vi "CRYSet Stimulus Editor Sub Front Panel.vi"(11 "Vi Ref":refnum<vi>) -> ()   [LabVIEW 2013]
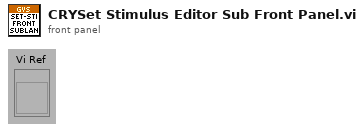
[diagram p1: front panel]
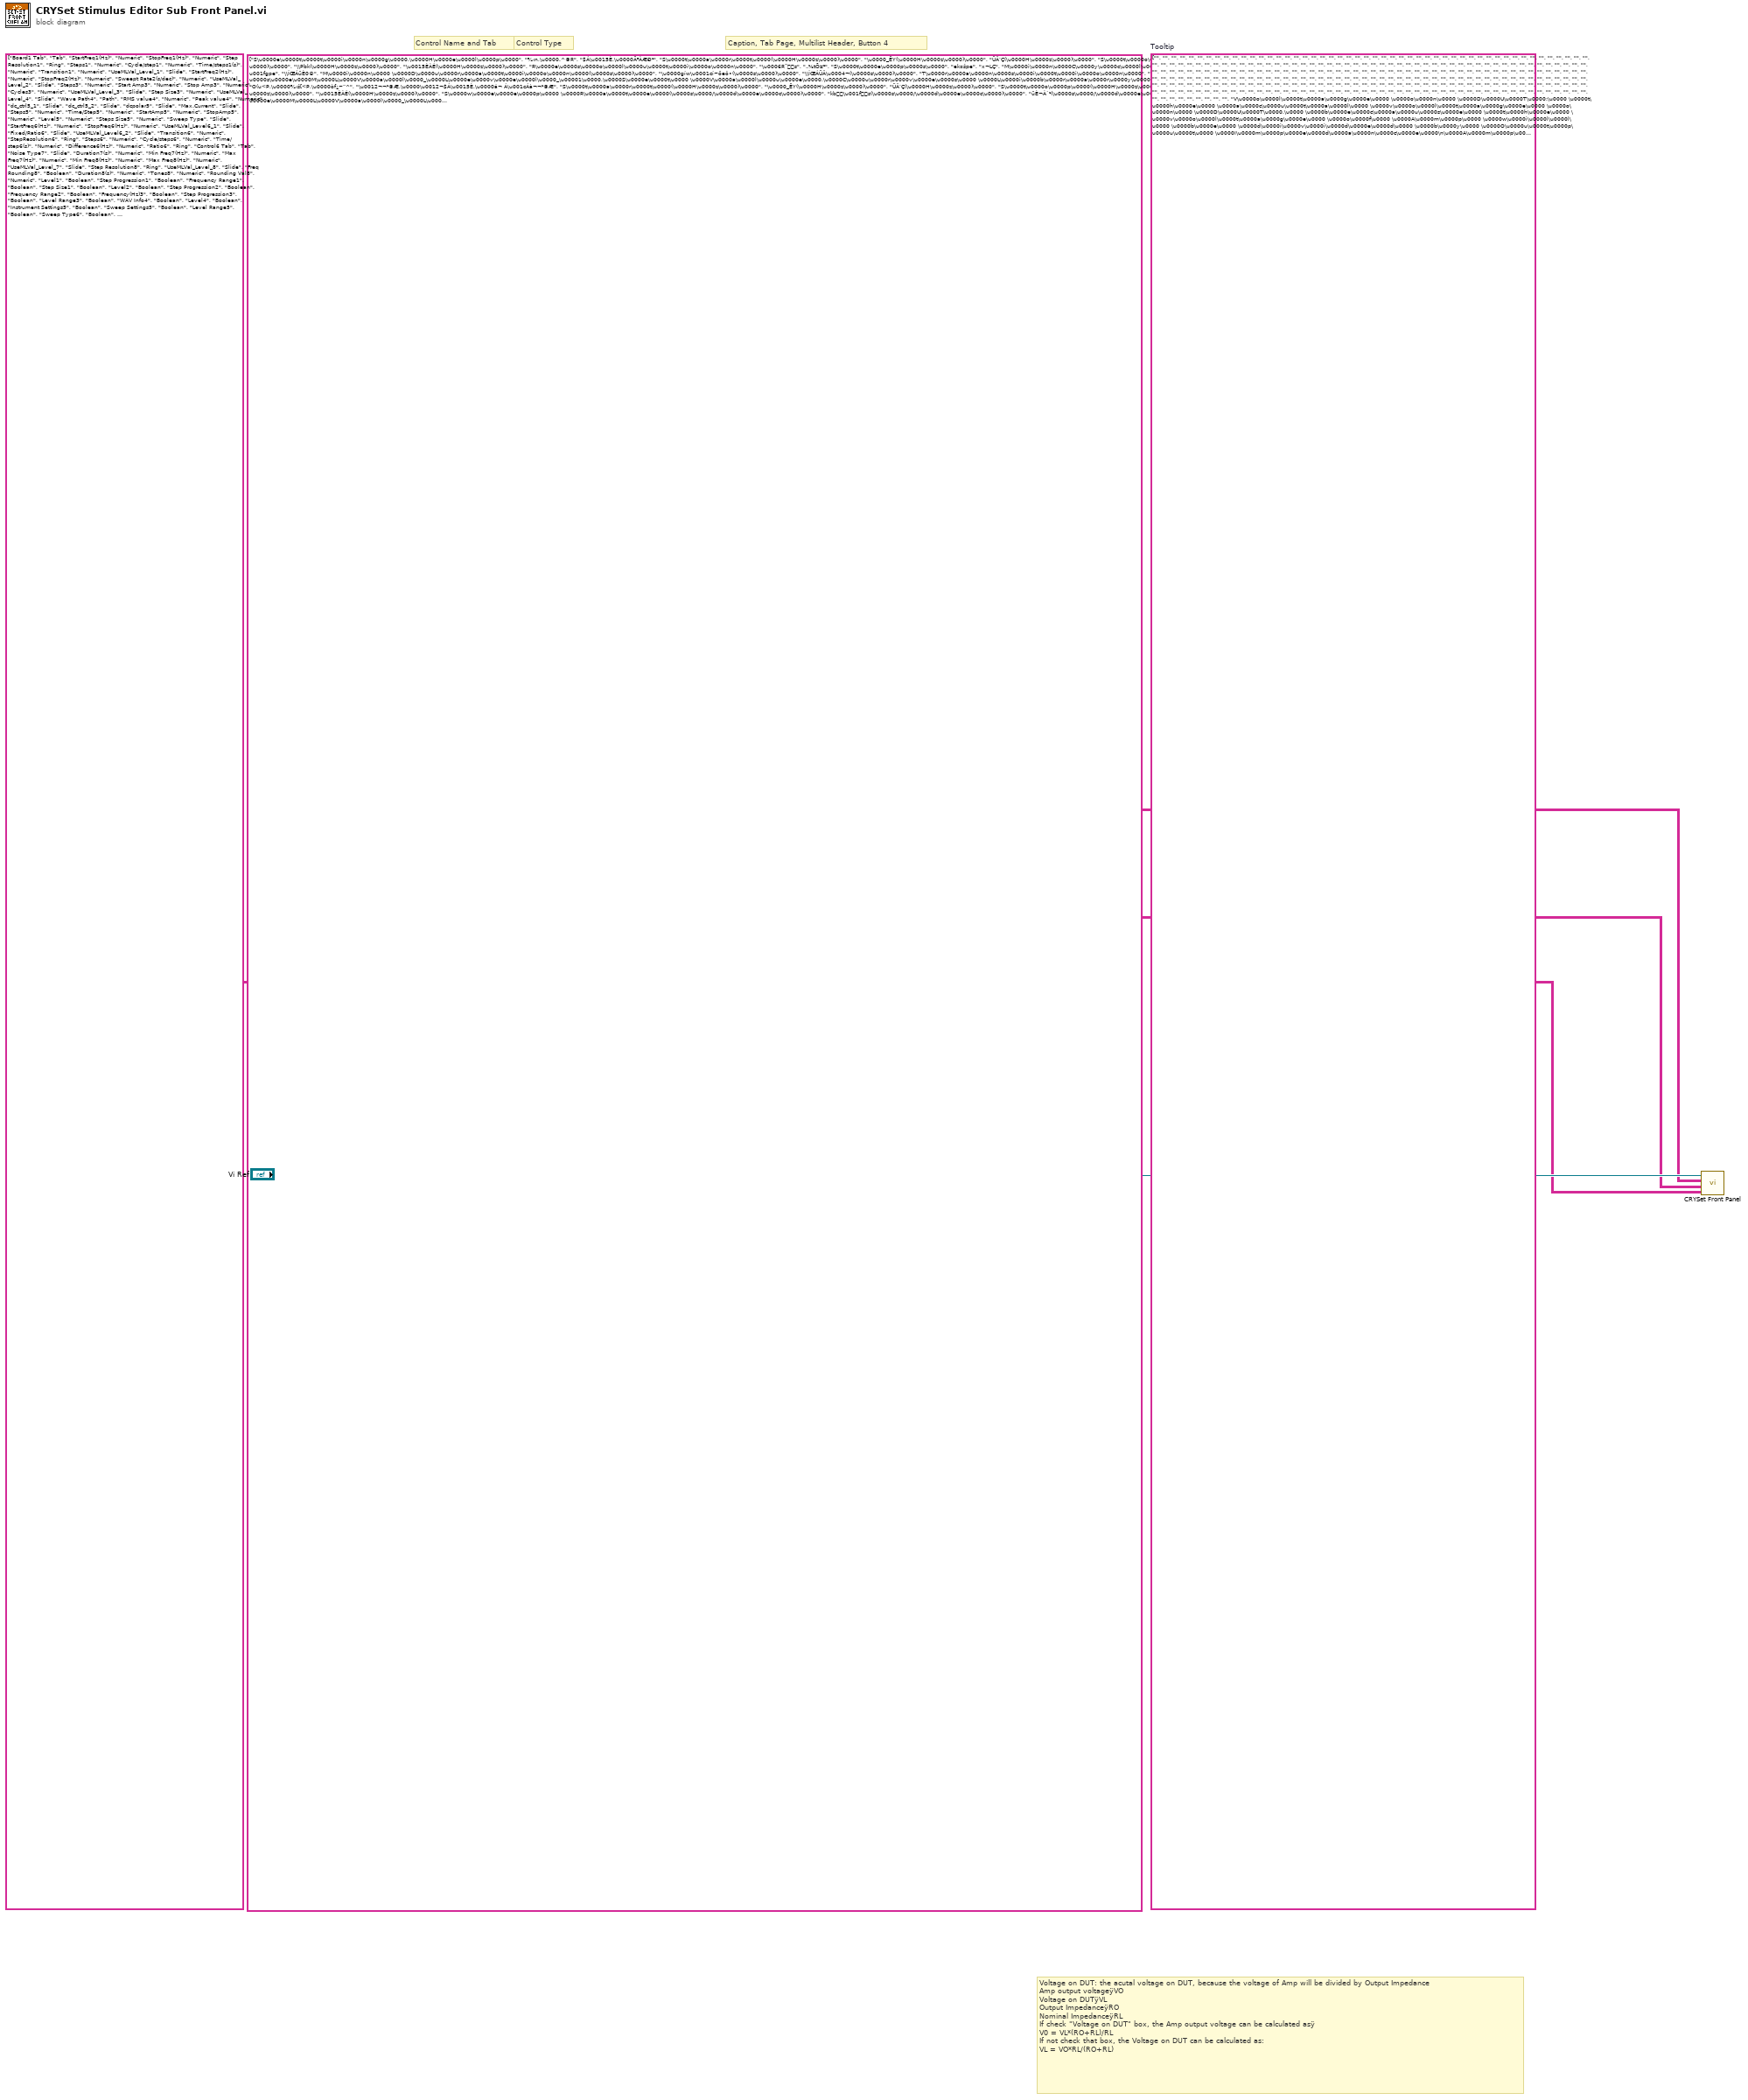
[diagram p0: block diagram]
diagram:
  w1 = string[][] [["", "", ""], ["", "", ""], ["", "", ""], ["", "", ""], ["", "", ""], ["", "", ""], ["", "", ""], ["", "", ""], ["", "", ""], ["", "", ""], ["", "", ""], ["", "", ""], ["", "", ""], ["", "", ""], ["", "", ""], ["", "", ""], ["", "", ""], ["", "", ""], ["", "", ""], ["", "", ""], ["", "", ""], ["", "", ""], ["", "", ""], ["", "", ""], ["", "", ""], ["", "", ""], ["", "", ""], ["", "", ""], ["", "", ""], ["", "", ""], ["", "", ""], ["", "", ""], ["", "", ""], ["", "", ""], ["", "", ""], ["", "", ""], ["", "", ""], ["", "", ""], ["", "", ""], ["", "", ""], ["", "", ""], ["", "", ""], ["", "", ""], ["", "", ""], ["", "", ""], ["", "", ""], ["", "", ""], ["", "", ""], ["", "", ""], ["", "", ""], ["", "", ""], ["", "", ""], ["", "", ""], ["", "", ""], ["", "", ""], ["", "", ""], ["", "", ""], ["", "", ""], ["", "", ""], ["", "", ""], ["", "", ""], ["", "", ""], ["", "", ""], ["", "", ""], ["", "", ""], ["", "", ""], ["", "", ""], ["", "", ""], ["", "", ""], ["", "", ""], ["", "", ""], ["", "", ""], ["", "", ""], ["", "", ""], ["", "", ""], ["", "", ""], ["", "", ""], ["", "", ""], ["", "", ""], ["", "", ""], ["", "", ""], ["", "", ""], ["", "", ""], ["", "", ""], ["", "", ""], ["", "", ""], ["", "", ""], ["", "", ""], ["", "", ""], ["", "", ""], ["", "", ""], ["", "", ""], ["", "", ""], ["", "", ""], ["", "", ""], ["", "", ""], ["", "", ""], ["", "", ""], ["", "", ""], ["", "", ""], ["", "", ""], ["", "", ""], ["", "", ""], ["V\u0000o\u0000l\u0000t\u0000a\u0000g\u0000e\u0000 \u0000o\u0000n\u0000 \u0000D\u0000U\u0000T\u0000:\u0000 \u0000t\u0000h\u0000e\u0000 \u0000a\u0000c\u0000u\u0000t\u0000a\u0000l\u0000 \u0000v\u0000o\u0000l\u0000t\u0000a\u0000g\u0000e\u0000 \u0000o\u0000n\u0000 \u0000D\u0000U\u0000T\u0000,\u0000 \u0000b\u0000e\u0000c\u0000a\u0000u\u0000s\u0000e\u0000 \u0000t\u0000h\u0000e\u0000 \u0000v\u0000o\u0000l\u0000t\u0000a\u0000g\u0000e\u0000 \u0000o\u0000f\u0000 \u0000A\u0000m\u0000p\u0000 \u0000w\u0000i\u0000l\u0000l\u0000 \u0000b\u0000e\u0000 \u0000d\u0000i\u0000v\u0000i\u0000d\u0000e\u0000d\u0000 \u0000b\u0000y\u0000 \u0000O\u0000u\u0000t\u0000p\u0000u\u0000t\u0000 \u0000I\u0000m\u0000p\u0000e\u0000d\u0000a\u0000n\u0000c\u0000e\u0000\n\u0000A\u0000m\u0000p\u0000 \u0000o\u0000u\u0000t\u0000p\u0000u\u0000t\u0000 \u0000v\u0000o\u0000l\u0000t\u0000a\u0000g\u0000e\u0000\u001aÿV\u0000O\u0000\n\u0000V\u0000o\u0000l\u0000t\u0000a\u0000g\u0000e\u0000 \u0000o\u0000n\u0000 \u0000D\u0000U\u0000T\u0000\u001aÿV\u0000L\u0000\n\u0000O\u0000u\u0000t\u0000p\u0000u\u0000t\u0000 \u0000I\u0000m\u0000p\u0000e\u0000d\u0000a\u0000n\u0000c\u0000e\u0000\u001aÿR\u0000O\u0000\n\u0000N\u0000o\u0000m\u0000i\u0000n\u0000a\u0000l\u0000 \u0000I\u0000m\u0000p\u0000e\u0000d\u0000a\u0000n\u0000c\u0000e\u0000\u001aÿR\u0000L\u0000\n\u0000I\u0000f\u0000 \u0000c\u0000h\u0000e\u0000c\u0000k\u0000 \u0000\"\u0000V\u0000o\u0000l\u0000t\u0000a\u0000g\u0000e\u0000 \u0000o\u0000n\u0000 \u0000D\u0000U\u0000T\u0000\"\u0000 \u0000b\u0000o\u0000x\u0000,\u0000 \u0000t\u0000h\u0000e\u0000 \u0000A\u0000m\u0000p\u0000 \u0000o\u0000u\u0000t\u0000p\u0000u\u0000t\u0000 \u0000v\u0000o\u0000l\u0000t\u0000a\u0000g\u0000e\u0000 \u0000c\u0000a\u0000n\u0000 \u0000b\u0000e\u0000 \u0000c\u0000a\u0000l\u0000c\u0000u\u0000l\u0000a\u0000t\u0000e\u0000d\u0000 \u0000a\u0000s\u0000\u001aÿ\n\u0000V\u00000\u0000 \u0000=\u0000 \u0000V\u0000L\u0000*\u0000(\u0000R\u0000O\u0000+\u0000R\u0000L\u0000)\u0000/\u0000R\u0000L\u0000\n\u0000I\u0000f\u0000 \u0000n\u0000o\u0000t\u0000 \u0000c\u0000h\u0000e\u0000c\u0000k\u0000 \u0000t\u0000h\u0000a\u0000t\u0000 \u0000...", "hVöN$Nïz5uS\u001aÿR>eúQv5uS\fÿÏ~ÇúQ;b\u0006RS\u000eT\fÿ(W«KmhVöN$Nïzv[E5uS\u00020\n\u0000\n\u0000R>eúQ5uS\u001aÿV\u0000O\u0000\n\u0000hVöN$Nïz5uS\u001aÿV\u0000L\u0000\n\u0000úQ;b\u001aÿR\u0000O\u0000\n\u0000\u0007hðy;b\u001aÿR\u0000L\u0000\n\u0000\n\u0000å\t-NhVöN$Nïz5uS\fÿ\u0019RR>eúQ5uS:N\u001aÿ\n\u0000V\u00000\u0000 \u0000=\u0000 \u0000V\u0000L\u0000*\u0000(\u0000R\u0000O\u0000+\u0000R\u0000L\u0000)\u0000/\u0000R\u0000L\u0000\n\u0000\n\u0000å\rN\t-N\fÿ\u0019RhVöN$Nïz5uS:N\u001aÿ\n\u0000V\u0000L\u0000 \u0000=\u0000 \u0000V\u0000O\u0000*\u0000R\u0000L\u0000/\u0000(\u0000R\u0000O\u0000+\u0000R\u0000L\u0000)\u0000", "V\u0000o\u0000l\u0000t\u0000a\u0000g\u0000e\u0000 \u0000o\u0000n\u0000 \u0000D\u0000U\u0000T\u0000:\u0000 \u0000t\u0000h\u0000e\u0000 \u0000a\u0000c\u0000u\u0000t\u0000a\u0000l\u0000 \u0000v\u0000o\u0000l\u0000t\u0000a\u0000g\u0000e\u0000 \u0000o\u0000n\u0000 \u0000D\u0000U\u0000T\u0000,\u0000 \u0000b\u0000e\u0000c\u0000a\u0000u\u0000s\u0000e\u0000 \u0000t\u0000h\u0000e\u0000 \u0000v\u0000o\u0000l\u0000t\u0000a\u0000g\u0000e\u0000 \u0000o\u0000f\u0000 \u0000A\u0000m\u0000p\u0000 \u0000w\u0000i\u0000l\u0000l\u0000 \u0000b\u0000e\u0000 \u0000d\u0000i\u0000v\u0000i\u0000d\u0000e\u0000d\u0000 \u0000b\u0000y\u0000 \u0000O\u0000u\u0000t\u0000p\u0000u\u0000t\u0000 \u0000I\u0000m\u0000p\u0000e\u0000d\u0000a\u0000n\u0000c\u0000e\u0000\n\u0000A\u0000m\u0000p\u0000 \u0000o\u0000u\u0000t\u0000p\u0000u\u0000t\u0000 \u0000v\u0000o\u0000l\u0000t\u0000a\u0000g\u0000e\u0000\u001aÿV\u0000O\u0000\n\u0000V\u0000o\u0000l\u0000t\u0000a\u0000g\u0000e\u0000 \u0000o\u0000n\u0000 \u0000D\u0000U\u0000T\u0000\u001aÿV\u0000L\u0000\n\u0000O\u0000u\u0000t\u0000p\u0000u\u0000t\u0000 \u0000I\u0000m\u0000p\u0000e\u0000d\u0000a\u0000n\u0000c\u0000e\u0000\u001aÿR\u0000O\u0000\n\u0000N\u0000o\u0000m\u0000i\u0000n\u0000a\u0000l\u0000 \u0000I\u0000m\u0000p\u0000e\u0000d\u0000a\u0000n\u0000c\u0000e\u0000\u001aÿR\u0000L\u0000\n\u0000I\u0000f\u0000 \u0000c\u0000h\u0000e\u0000c\u0000k\u0000 \u0000\"\u0000V\u0000o\u0000l\u0000t\u0000a\u0000g\u0000e\u0000 \u0000o\u0000n\u0000 \u0000D\u0000U\u0000T\u0000\"\u0000 \u0000b\u0000o\u0000x\u0000,\u0000 \u0000t\u0000h\u0000e\u0000 \u0000A\u0000m\u0000p\u0000 \u0000o\u0000u\u0000t\u0000p\u0000u\u0000t\u0000 \u0000v\u0000o\u0000l\u0000t\u0000a\u0000g\u0000e\u0000 \u0000c\u0000a\u0000n\u0000 \u0000b\u0000e\u0000 \u0000c\u0000a\u0000l\u0000c\u0000u\u0000l\u0000a\u0000t\u0000e\u0000d\u0000 \u0000a\u0000s\u0000\u001aÿ\n\u0000V\u00000\u0000 \u0000=\u0000 \u0000V\u0000L\u0000*\u0000(\u0000R\u0000O\u0000+\u0000R\u0000L\u0000)\u0000/\u0000R\u0000L\u0000\n\u0000I\u0000f\u0000 \u0000n\u0000o\u0000t\u0000 \u0000c\u0000h\u0000e\u0000c\u0000k\u0000 \u0000t\u0000h\u0000a\u0000t\u0000 \u0000..."], ["", "", ""], ["", "", ""], ["V\u0000o\u0000l\u0000t\u0000a\u0000g\u0000e\u0000 \u0000o\u0000n\u0000 \u0000D\u0000U\u0000T\u0000:\u0000 \u0000t\u0000h\u0000e\u0000 \u0000a\u0000c\u0000u\u0000t\u0000a\u0000l\u0000 \u0000v\u0000o\u0000l\u0000t\u0000a\u0000g\u0000e\u0000 \u0000o\u0000n\u0000 \u0000D\u0000U\u0000T\u0000,\u0000 \u0000b\u0000e\u0000c\u0000a\u0000u\u0000s\u0000e\u0000 \u0000t\u0000h\u0000e\u0000 \u0000v\u0000o\u0000l\u0000t\u0000a\u0000g\u0000e\u0000 \u0000o\u0000f\u0000 \u0000A\u0000m\u0000p\u0000 \u0000w\u0000i\u0000l\u0000l\u0000 \u0000b\u0000e\u0000 \u0000d\u0000i\u0000v\u0000i\u0000d\u0000e\u0000d\u0000 \u0000b\u0000y\u0000 \u0000O\u0000u\u0000t\u0000p\u0000u\u0000t\u0000 \u0000I\u0000m\u0000p\u0000e\u0000d\u0000a\u0000n\u0000c\u0000e\u0000\n\u0000A\u0000m\u0000p\u0000 \u0000o\u0000u\u0000t\u0000p\u0000u\u0000t\u0000 \u0000v\u0000o\u0000l\u0000t\u0000a\u0000g\u0000e\u0000\u001aÿV\u0000O\u0000\n\u0000V\u0000o\u0000l\u0000t\u0000a\u0000g\u0000e\u0000 \u0000o\u0000n\u0000 \u0000D\u0000U\u0000T\u0000\u001aÿV\u0000L\u0000\n\u0000O\u0000u\u0000t\u0000p\u0000u\u0000t\u0000 \u0000I\u0000m\u0000p\u0000e\u0000d\u0000a\u0000n\u0000c\u0000e\u0000\u001aÿR\u0000O\u0000\n\u0000N\u0000o\u0000m\u0000i\u0000n\u0000a\u0000l\u0000 \u0000I\u0000m\u0000p\u0000e\u0000d\u0000a\u0000n\u0000c\u0000e\u0000\u001aÿR\u0000L\u0000\n\u0000I\u0000f\u0000 \u0000c\u0000h\u0000e\u0000c\u0000k\u0000 \u0000\"\u0000V\u0000o\u0000l\u0000t\u0000a\u0000g\u0000e\u0000 \u0000o\u0000n\u0000 \u0000D\u0000U\u0000T\u0000\"\u0000 \u0000b\u0000o\u0000x\u0000,\u0000 \u0000t\u0000h\u0000e\u0000 \u0000A\u0000m\u0000p\u0000 \u0000o\u0000u\u0000t\u0000p\u0000u\u0000t\u0000 \u0000v\u0000o\u0000l\u0000t\u0000a\u0000g\u0000e\u0000 \u0000c\u0000a\u0000n\u0000 \u0000b\u0000e\u0000 \u0000c\u0000a\u0000l\u0000c\u0000u\u0000l\u0000a\u0000t\u0000e\u0000d\u0000 \u0000a\u0000s\u0000\u001aÿ\n\u0000V\u00000\u0000 \u0000=\u0000 \u0000V\u0000L\u0000*\u0000(\u0000R\u0000O\u0000+\u0000R\u0000L\u0000)\u0000/\u0000R\u0000L\u0000\n\u0000I\u0000f\u0000 \u0000n\u0000o\u0000t\u0000 \u0000c\u0000h\u0000e\u0000c\u0000k\u0000 \u0000t\u0000h\u0000a\u0000t\u0000 \u0000...", "hVöN$Nïz5uS\u001aÿR>eúQv5uS\fÿÏ~ÇúQ;b\u0006RS\u000eT\fÿ(W«KmhVöN$Nïzv[E5uS\u00020\n\u0000\n\u0000R>eúQ5uS\u001aÿV\u0000O\u0000\n\u0000hVöN$Nïz5uS\u001aÿV\u0000L\u0000\n\u0000úQ;b\u001aÿR\u0000O\u0000\n\u0000\u0007hðy;b\u001aÿR\u0000L\u0000\n\u0000\n\u0000å\t-NhVöN$Nïz5uS\fÿ\u0019RR>eúQ5uS:N\u001aÿ\n\u0000V\u00000\u0000 \u0000=\u0000 \u0000V\u0000L\u0000*\u0000(\u0000R\u0000O\u0000+\u0000R\u0000L\u0000)\u0000/\u0000R\u0000L\u0000\n\u0000\n\u0000å\rN\t-N\fÿ\u0019RhVöN$Nïz5uS:N\u001aÿ\n\u0000V\u0000L\u0000 \u0000=\u0000 \u0000V\u0000O\u0000*\u0000R\u0000L\u0000/\u0000(\u0000R\u0000O\u0000+\u0000R\u0000L\u0000)\u0000", "V\u0000o\u0000l\u0000t\u0000a\u0000g\u0000e\u0000 \u0000o\u0000n\u0000 \u0000D\u0000U\u0000T\u0000:\u0000 \u0000t\u0000h\u0000e\u0000 \u0000a\u0000c\u0000u\u0000t\u0000a\u0000l\u0000 \u0000v\u0000o\u0000l\u0000t\u0000a\u0000g\u0000e\u0000 \u0000o\u0000n\u0000 \u0000D\u0000U\u0000T\u0000,\u0000 \u0000b\u0000e\u0000c\u0000a\u0000u\u0000s\u0000e\u0000 \u0000t\u0000h\u0000e\u0000 \u0000v\u0000o\u0000l\u0000t\u0000a\u0000g\u0000e\u0000 \u0000o\u0000f\u0000 \u0000A\u0000m\u0000p\u0000 \u0000w\u0000i\u0000l\u0000l\u0000 \u0000b\u0000e\u0000 \u0000d\u0000i\u0000v\u0000i\u0000d\u0000e\u0000d\u0000 \u0000b\u0000y\u0000 \u0000O\u0000u\u0000t\u0000p\u0000u\u0000t\u0000 \u0000I\u0000m\u0000p\u0000e\u0000d\u0000a\u0000n\u0000c\u0000e\u0000\n\u0000A\u0000m\u0000p\u0000 \u0000o\u0000u\u0000t\u0000p\u0000u\u0000t\u0000 \u0000v\u0000o\u0000l\u0000t\u0000a\u0000g\u0000e\u0000\u001aÿV\u0000O\u0000\n\u0000V\u0000o\u0000l\u0000t\u0000a\u0000g\u0000e\u0000 \u0000o\u0000n\u0000 \u0000D\u0000U\u0000T\u0000\u001aÿV\u0000L\u0000\n\u0000O\u0000u\u0000t\u0000p\u0000u\u0000t\u0000 \u0000I\u0000m\u0000p\u0000e\u0000d\u0000a\u0000n\u0000c\u0000e\u0000\u001aÿR\u0000O\u0000\n\u0000N\u0000o\u0000m\u0000i\u0000n\u0000a\u0000l\u0000 \u0000I\u0000m\u0000p\u0000e\u0000d\u0000a\u0000n\u0000c\u0000e\u0000\u001aÿR\u0000L\u0000\n\u0000I\u0000f\u0000 \u0000c\u0000h\u0000e\u0000c\u0000k\u0000 \u0000\"\u0000V\u0000o\u0000l\u0000t\u0000a\u0000g\u0000e\u0000 \u0000o\u0000n\u0000 \u0000D\u0000U\u0000T\u0000\"\u0000 \u0000b\u0000o\u0000x\u0000,\u0000 \u0000t\u0000h\u0000e\u0000 \u0000A\u0000m\u0000p\u0000 \u0000o\u0000u\u0000t\u0000p\u0000u\u0000t\u0000 \u0000v\u0000o\u0000l\u0000t\u0000a\u0000g\u0000e\u0000 \u0000c\u0000a\u0000n\u0000 \u0000b\u0000e\u0000 \u0000c\u0000a\u0000l\u0000c\u0000u\u0000l\u0000a\u0000t\u0000e\u0000d\u0000 \u0000a\u0000s\u0000\u001aÿ\n\u0000V\u00000\u0000 \u0000=\u0000 \u0000V\u0000L\u0000*\u0000(\u0000R\u0000O\u0000+\u0000R\u0000L\u0000)\u0000/\u0000R\u0000L\u0000\n\u0000I\u0000f\u0000 \u0000n\u0000o\u0000t\u0000 \u0000c\u0000h\u0000e\u0000c\u0000k\u0000 \u0000t\u0000h\u0000a\u0000t\u0000 \u0000..."], ["", "", ""], ["", "", ""], ["V\u0000o\u0000l\u0000t\u0000a\u0000g\u0000e\u0000 \u0000o\u0000n\u0000 \u0000D\u0000U\u0000T\u0000:\u0000 \u0000t\u0000h\u0000e\u0000 \u0000a\u0000c\u0000u\u0000t\u0000a\u0000l\u0000 \u0000v\u0000o\u0000l\u0000t\u0000a\u0000g\u0000e\u0000 \u0000o\u0000n\u0000 \u0000D\u0000U\u0000T\u0000,\u0000 \u0000b\u0000e\u0000c\u0000a\u0000u\u0000s\u0000e\u0000 \u0000t\u0000h\u0000e\u0000 \u0000v\u0000o\u0000l\u0000t\u0000a\u0000g\u0000e\u0000 \u0000o\u0000f\u0000 \u0000A\u0000m\u0000p\u0000 \u0000w\u0000i\u0000l\u0000l\u0000 \u0000b\u0000e\u0000 \u0000d\u0000i\u0000v\u0000i\u0000d\u0000e\u0000d\u0000 \u0000b\u0000y\u0000 \u0000O\u0000u\u0000t\u0000p\u0000u\u0000t\u0000 \u0000I\u0000m\u0000p\u0000e\u0000d\u0000a\u0000n\u0000c\u0000e\u0000\n\u0000A\u0000m\u0000p\u0000 \u0000o\u0000u\u0000t\u0000p\u0000u\u0000t\u0000 \u0000v\u0000o\u0000l\u0000t\u0000a\u0000g\u0000e\u0000\u001aÿV\u0000O\u0000\n\u0000V\u0000o\u0000l\u0000t\u0000a\u0000g\u0000e\u0000 \u0000o\u0000n\u0000 \u0000D\u0000U\u0000T\u0000\u001aÿV\u0000L\u0000\n\u0000O\u0000u\u0000t\u0000p\u0000u\u0000t\u0000 \u0000I\u0000m\u0000p\u0000e\u0000d\u0000a\u0000n\u0000c\u0000e\u0000\u001aÿR\u0000O\u0000\n\u0000N\u0000o\u0000m\u0000i\u0000n\u0000a\u0000l\u0000 \u0000I\u0000m\u0000p\u0000e\u0000d\u0000a\u0000n\u0000c\u0000e\u0000\u001aÿR\u0000L\u0000\n\u0000I\u0000f\u0000 \u0000c\u0000h\u0000e\u0000c\u0000k\u0000 \u0000\"\u0000V\u0000o\u0000l\u0000t\u0000a\u0000g\u0000e\u0000 \u0000o\u0000n\u0000 \u0000D\u0000U\u0000T\u0000\"\u0000 \u0000b\u0000o\u0000x\u0000,\u0000 \u0000t\u0000h\u0000e\u0000 \u0000A\u0000m\u0000p\u0000 \u0000o\u0000u\u0000t\u0000p\u0000u\u0000t\u0000 \u0000v\u0000o\u0000l\u0000t\u0000a\u0000g\u0000e\u0000 \u0000c\u0000a\u0000n\u0000 \u0000b\u0000e\u0000 \u0000c\u0000a\u0000l\u0000c\u0000u\u0000l\u0000a\u0000t\u0000e\u0000d\u0000 \u0000a\u0000s\u0000\u001aÿ\n\u0000V\u00000\u0000 \u0000=\u0000 \u0000V\u0000L\u0000*\u0000(\u0000R\u0000O\u0000+\u0000R\u0000L\u0000)\u0000/\u0000R\u0000L\u0000\n\u0000I\u0000f\u0000 \u0000n\u0000o\u0000t\u0000 \u0000c\u0000h\u0000e\u0000c\u0000k\u0000 \u0000t\u0000h\u0000a\u0000t\u0000 \u0000...", "hVöN$Nïz5uS\u001aÿR>eúQv5uS\fÿÏ~ÇúQ;b\u0006RS\u000eT\fÿ(W«KmhVöN$Nïzv[E5uS\u00020\n\u0000\n\u0000R>eúQ5uS\u001aÿV\u0000O\u0000\n\u0000hVöN$Nïz5uS\u001aÿV\u0000L\u0000\n\u0000úQ;b\u001aÿR\u0000O\u0000\n\u0000\u0007hðy;b\u001aÿR\u0000L\u0000\n\u0000\n\u0000å\t-NhVöN$Nïz5uS\fÿ\u0019RR>eúQ5uS:N\u001aÿ\n\u0000V\u00000\u0000 \u0000=\u0000 \u0000V\u0000L\u0000*\u0000(\u0000R\u0000O\u0000+\u0000R\u0000L\u0000)\u0000/\u0000R\u0000L\u0000\n\u0000\n\u0000å\rN\t-N\fÿ\u0019RhVöN$Nïz5uS:N\u001aÿ\n\u0000V\u0000L\u0000 \u0000=\u0000 \u0000V\u0000O\u0000*\u0000R\u0000L\u0000/\u0000(\u0000R\u0000O\u0000+\u0000R\u0000L\u0000)\u0000", "V\u0000o\u0000l\u0000t\u0000a\u0000g\u0000e\u0000 \u0000o\u0000n\u0000 \u0000D\u0000U\u0000T\u0000:\u0000 \u0000t\u0000h\u0000e\u0000 \u0000a\u0000c\u0000u\u0000t\u0000a\u0000l\u0000 \u0000v\u0000o\u0000l\u0000t\u0000a\u0000g\u0000e\u0000 \u0000o\u0000n\u0000 \u0000D\u0000U\u0000T\u0000,\u0000 \u0000b\u0000e\u0000c\u0000a\u0000u\u0000s\u0000e\u0000 \u0000t\u0000h\u0000e\u0000 \u0000v\u0000o\u0000l\u0000t\u0000a\u0000g\u0000e\u0000 \u0000o\u0000f\u0000 \u0000A\u0000m\u0000p\u0000 \u0000w\u0000i\u0000l\u0000l\u0000 \u0000b\u0000e\u0000 \u0000d\u0000i\u0000v\u0000i\u0000d\u0000e\u0000d\u0000 \u0000b\u0000y\u0000 \u0000O\u0000u\u0000t\u0000p\u0000u\u0000t\u0000 \u0000I\u0000m\u0000p\u0000e\u0000d\u0000a\u0000n\u0000c\u0000e\u0000\n\u0000A\u0000m\u0000p\u0000 \u0000o\u0000u\u0000t\u0000p\u0000u\u0000t\u0000 \u0000v\u0000o\u0000l\u0000t\u0000a\u0000g\u0000e\u0000\u001aÿV\u0000O\u0000\n\u0000V\u0000o\u0000l\u0000t\u0000a\u0000g\u0000e\u0000 \u0000o\u0000n\u0000 \u0000D\u0000U\u0000T\u0000\u001aÿV\u0000L\u0000\n\u0000O\u0000u\u0000t\u0000p\u0000u\u0000t\u0000 \u0000I\u0000m\u0000p\u0000e\u0000d\u0000a\u0000n\u0000c\u0000e\u0000\u001aÿR\u0000O\u0000\n\u0000N\u0000o\u0000m\u0000i\u0000n\u0000a\u0000l\u0000 \u0000I\u0000m\u0000p\u0000e\u0000d\u0000a\u0000n\u0000c\u0000e\u0000\u001aÿR\u0000L\u0000\n\u0000I\u0000f\u0000 \u0000c\u0000h\u0000e\u0000c\u0000k\u0000 \u0000\"\u0000V\u0000o\u0000l\u0000t\u0000a\u0000g\u0000e\u0000 \u0000o\u0000n\u0000 \u0000D\u0000U\u0000T\u0000\"\u0000 \u0000b\u0000o\u0000x\u0000,\u0000 \u0000t\u0000h\u0000e\u0000 \u0000A\u0000m\u0000p\u0000 \u0000o\u0000u\u0000t\u0000p\u0000u\u0000t\u0000 \u0000v\u0000o\u0000l\u0000t\u0000a\u0000g\u0000e\u0000 \u0000c\u0000a\u0000n\u0000 \u0000b\u0000e\u0000 \u0000c\u0000a\u0000l\u0000c\u0000u\u0000l\u0000a\u0000t\u0000e\u0000d\u0000 \u0000a\u0000s\u0000\u001aÿ\n\u0000V\u00000\u0000 \u0000=\u0000 \u0000V\u0000L\u0000*\u0000(\u0000R\u0000O\u0000+\u0000R\u0000L\u0000)\u0000/\u0000R\u0000L\u0000\n\u0000I\u0000f\u0000 \u0000n\u0000o\u0000t\u0000 \u0000c\u0000h\u0000e\u0000c\u0000k\u0000 \u0000t\u0000h\u0000a\u0000t\u0000 \u0000..."], ["", "", ""], ["", "", ""], ["V\u0000o\u0000l\u0000t\u0000a\u0000g\u0000e\u0000 \u0000o\u0000n\u0000 \u0000D\u0000U\u0000T\u0000:\u0000 \u0000t\u0000h\u0000e\u0000 \u0000a\u0000c\u0000u\u0000t\u0000a\u0000l\u0000 \u0000v\u0000o\u0000l\u0000t\u0000a\u0000g\u0000e\u0000 \u0000o\u0000n\u0000 \u0000D\u0000U\u0000T\u0000,\u0000 \u0000b\u0000e\u0000c\u0000a\u0000u\u0000s\u0000e\u0000 \u0000t\u0000h\u0000e\u0000 \u0000v\u0000o\u0000l\u0000t\u0000a\u0000g\u0000e\u0000 \u0000o\u0000f\u0000 \u0000A\u0000m\u0000p\u0000 \u0000w\u0000i\u0000l\u0000l\u0000 \u0000b\u0000e\u0000 \u0000d\u0000i\u0000v\u0000i\u0000d\u0000e\u0000d\u0000 \u0000b\u0000y\u0000 \u0000O\u0000u\u0000t\u0000p\u0000u\u0000t\u0000 \u0000I\u0000m\u0000p\u0000e\u0000d\u0000a\u0000n\u0000c\u0000e\u0000\n\u0000A\u0000m\u0000p\u0000 \u0000o\u0000u\u0000t\u0000p\u0000u\u0000t\u0000 \u0000v\u0000o\u0000l\u0000t\u0000a\u0000g\u0000e\u0000\u001aÿV\u0000O\u0000\n\u0000V\u0000o\u0000l\u0000t\u0000a\u0000g\u0000e\u0000 \u0000o\u0000n\u0000 \u0000D\u0000U\u0000T\u0000\u001aÿV\u0000L\u0000\n\u0000O\u0000u\u0000t\u0000p\u0000u\u0000t\u0000 \u0000I\u0000m\u0000p\u0000e\u0000d\u0000a\u0000n\u0000c\u0000e\u0000\u001aÿR\u0000O\u0000\n\u0000N\u0000o\u0000m\u0000i\u0000n\u0000a\u0000l\u0000 \u0000I\u0000m\u0000p\u0000e\u0000d\u0000a\u0000n\u0000c\u0000e\u0000\u001aÿR\u0000L\u0000\n\u0000I\u0000f\u0000 \u0000c\u0000h\u0000e\u0000c\u0000k\u0000 \u0000\"\u0000V\u0000o\u0000l\u0000t\u0000a\u0000g\u0000e\u0000 \u0000o\u0000n\u0000 \u0000D\u0000U\u0000T\u0000\"\u0000 \u0000b\u0000o\u0000x\u0000,\u0000 \u0000t\u0000h\u0000e\u0000 \u0000A\u0000m\u0000p\u0000 \u0000o\u0000u\u0000t\u0000p\u0000u\u0000t\u0000 \u0000v\u0000o\u0000l\u0000t\u0000a\u0000g\u0000e\u0000 \u0000c\u0000a\u0000n\u0000 \u0000b\u0000e\u0000 \u0000c\u0000a\u0000l\u0000c\u0000u\u0000l\u0000a\u0000t\u0000e\u0000d\u0000 \u0000a\u0000s\u0000\u001aÿ\n\u0000V\u00000\u0000 \u0000=\u0000 \u0000V\u0000L\u0000*\u0000(\u0000R\u0000O\u0000+\u0000R\u0000L\u0000)\u0000/\u0000R\u0000L\u0000\n\u0000I\u0000f\u0000 \u0000n\u0000o\u0000t\u0000 \u0000c\u0000h\u0000e\u0000c\u0000k\u0000 \u0000t\u0000h\u0000a\u0000t\u0000 \u0000...", "hVöN$Nïz5uS\u001aÿR>eúQv5uS\fÿÏ~ÇúQ;b\u0006RS\u000eT\fÿ(W«KmhVöN$Nïzv[E5uS\u00020\n\u0000\n\u0000R>eúQ5uS\u001aÿV\u0000O\u0000\n\u0000hVöN$Nïz5uS\u001aÿV\u0000L\u0000\n\u0000úQ;b\u001aÿR\u0000O\u0000\n\u0000\u0007hðy;b\u001aÿR\u0000L\u0000\n\u0000\n\u0000å\t-NhVöN$Nïz5uS\fÿ\u0019RR>eúQ5uS:N\u001aÿ\n\u0000V\u00000\u0000 \u0000=\u0000 \u0000V\u0000L\u0000*\u0000(\u0000R\u0000O\u0000+\u0000R\u0000L\u0000)\u0000/\u0000R\u0000L\u0000\n\u0000\n\u0000å\rN\t-N\fÿ\u0019RhVöN$Nïz5uS:N\u001aÿ\n\u0000V\u0000L\u0000 \u0000=\u0000 \u0000V\u0000O\u0000*\u0000R\u0000L\u0000/\u0000(\u0000R\u0000O\u0000+\u0000R\u0000L\u0000)\u0000", "V\u0000o\u0000l\u0000t\u0000a\u0000g\u0000e\u0000 \u0000o\u0000n\u0000 \u0000D\u0000U\u0000T\u0000:\u0000 \u0000t\u0000h\u0000e\u0000 \u0000a\u0000c\u0000u\u0000t\u0000a\u0000l\u0000 \u0000v\u0000o\u0000l\u0000t\u0000a\u0000g\u0000e\u0000 \u0000o\u0000n\u0000 \u0000D\u0000U\u0000T\u0000,\u0000 \u0000b\u0000e\u0000c\u0000a\u0000u\u0000s\u0000e\u0000 \u0000t\u0000h\u0000e\u0000 \u0000v\u0000o\u0000l\u0000t\u0000a\u0000g\u0000e\u0000 \u0000o\u0000f\u0000 \u0000A\u0000m\u0000p\u0000 \u0000w\u0000i\u0000l\u0000l\u0000 \u0000b\u0000e\u0000 \u0000d\u0000i\u0000v\u0000i\u0000d\u0000e\u0000d\u0000 \u0000b\u0000y\u0000 \u0000O\u0000u\u0000t\u0000p\u0000u\u0000t\u0000 \u0000I\u0000m\u0000p\u0000e\u0000d\u0000a\u0000n\u0000c\u0000e\u0000\n\u0000A\u0000m\u0000p\u0000 \u0000o\u0000u\u0000t\u0000p\u0000u\u0000t\u0000 \u0000v\u0000o\u0000l\u0000t\u0000a\u0000g\u0000e\u0000\u001aÿV\u0000O\u0000\n\u0000V\u0000o\u0000l\u0000t\u0000a\u0000g\u0000e\u0000 \u0000o\u0000n\u0000 \u0000D\u0000U\u0000T\u0000\u001aÿV\u0000L\u0000\n\u0000O\u0000u\u0000t\u0000p\u0000u\u0000t\u0000 \u0000I\u0000m\u0000p\u0000e\u0000d\u0000a\u0000n\u0000c\u0000e\u0000\u001aÿR\u0000O\u0000\n\u0000N\u0000o\u0000m\u0000i\u0000n\u0000a\u0000l\u0000 \u0000I\u0000m\u0000p\u0000e\u0000d\u0000a\u0000n\u0000c\u0000e\u0000\u001aÿR\u0000L\u0000\n\u0000I\u0000f\u0000 \u0000c\u0000h\u0000e\u0000c\u0000k\u0000 \u0000\"\u0000V\u0000o\u0000l\u0000t\u0000a\u0000g\u0000e\u0000 \u0000o\u0000n\u0000 \u0000D\u0000U\u0000T\u0000\"\u0000 \u0000b\u0000o\u0000x\u0000,\u0000 \u0000t\u0000h\u0000e\u0000 \u0000A\u0000m\u0000p\u0000 \u0000o\u0000u\u0000t\u0000p\u0000u\u0000t\u0000 \u0000v\u0000o\u0000l\u0000t\u0000a\u0000g\u0000e\u0000 \u0000c\u0000a\u0000n\u0000 \u0000b\u0000e\u0000 \u0000c\u0000a\u0000l\u0000c\u0000u\u0000l\u0000a\u0000t\u0000e\u0000d\u0000 \u0000a\u0000s\u0000\u001aÿ\n\u0000V\u00000\u0000 \u0000=\u0000 \u0000V\u0000L\u0000*\u0000(\u0000R\u0000O\u0000+\u0000R\u0000L\u0000)\u0000/\u0000R\u0000L\u0000\n\u0000I\u0000f\u0000 \u0000n\u0000o\u0000t\u0000 \u0000c\u0000h\u0000e\u0000c\u0000k\u0000 \u0000t\u0000h\u0000a\u0000t\u0000 \u0000..."], ["", "", ""], ["", "", ""], ["V\u0000o\u0000l\u0000t\u0000a\u0000g\u0000e\u0000 \u0000o\u0000n\u0000 \u0000D\u0000U\u0000T\u0000:\u0000 \u0000t\u0000h\u0000e\u0000 \u0000a\u0000c\u0000u\u0000t\u0000a\u0000l\u0000 \u0000v\u0000o\u0000l\u0000t\u0000a\u0000g\u0000e\u0000 \u0000o\u0000n\u0000 \u0000D\u0000U\u0000T\u0000,\u0000 \u0000b\u0000e\u0000c\u0000a\u0000u\u0000s\u0000e\u0000 \u0000t\u0000h\u0000e\u0000 \u0000v\u0000o\u0000l\u0000t\u0000a\u0000g\u0000e\u0000 \u0000o\u0000f\u0000 \u0000A\u0000m\u0000p\u0000 \u0000w\u0000i\u0000l\u0000l\u0000 \u0000b\u0000e\u0000 \u0000d\u0000i\u0000v\u0000i\u0000d\u0000e\u0000d\u0000 \u0000b\u0000y\u0000 \u0000O\u0000u\u0000t\u0000p\u0000u\u0000t\u0000 \u0000I\u0000m\u0000p\u0000e\u0000d\u0000a\u0000n\u0000c\u0000e\u0000\n\u0000A\u0000m\u0000p\u0000 \u0000o\u0000u\u0000t\u0000p\u0000u\u0000t\u0000 \u0000v\u0000o\u0000l\u0000t\u0000a\u0000g\u0000e\u0000\u001aÿV\u0000O\u0000\n\u0000V\u0000o\u0000l\u0000t\u0000a\u0000g\u0000e\u0000 \u0000o\u0000n\u0000 \u0000D\u0000U\u0000T\u0000\u001aÿV\u0000L\u0000\n\u0000O\u0000u\u0000t\u0000p\u0000u\u0000t\u0000 \u0000I\u0000m\u0000p\u0000e\u0000d\u0000a\u0000n\u0000c\u0000e\u0000\u001aÿR\u0000O\u0000\n\u0000N\u0000o\u0000m\u0000i\u0000n\u0000a\u0000l\u0000 \u0000I\u0000m\u0000p\u0000e\u0000d\u0000a\u0000n\u0000c\u0000e\u0000\u001aÿR\u0000L\u0000\n\u0000I\u0000f\u0000 \u0000c\u0000h\u0000e\u0000c\u0000k\u0000 \u0000\"\u0000V\u0000o\u0000l\u0000t\u0000a\u0000g\u0000e\u0000 \u0000o\u0000n\u0000 \u0000D\u0000U\u0000T\u0000\"\u0000 \u0000b\u0000o\u0000x\u0000,\u0000 \u0000t\u0000h\u0000e\u0000 \u0000A\u0000m\u0000p\u0000 \u0000o\u0000u\u0000t\u0000p\u0000u\u0000t\u0000 \u0000v\u0000o\u0000l\u0000t\u0000a\u0000g\u0000e\u0000 \u0000c\u0000a\u0000n\u0000 \u0000b\u0000e\u0000 \u0000c\u0000a\u0000l\u0000c\u0000u\u0000l\u0000a\u0000t\u0000e\u0000d\u0000 \u0000a\u0000s\u0000\u001aÿ\n\u0000V\u00000\u0000 \u0000=\u0000 \u0000V\u0000L\u0000*\u0000(\u0000R\u0000O\u0000+\u0000R\u0000L\u0000)\u0000/\u0000R\u0000L\u0000\n\u0000I\u0000f\u0000 \u0000n\u0000o\u0000t\u0000 \u0000c\u0000h\u0000e\u0000c\u0000k\u0000 \u0000t\u0000h\u0000a\u0000t\u0000 \u0000...", "hVöN$Nïz5uS\u001aÿR>eúQv5uS\fÿÏ~ÇúQ;b\u0006RS\u000eT\fÿ(W«KmhVöN$Nïzv[E5uS\u00020\n\u0000\n\u0000R>eúQ5uS\u001aÿV\u0000O\u0000\n\u0000hVöN$Nïz5uS\u001aÿV\u0000L\u0000\n\u0000úQ;b\u001aÿR\u0000O\u0000\n\u0000\u0007hðy;b\u001aÿR\u0000L\u0000\n\u0000\n\u0000å\t-NhVöN$Nïz5uS\fÿ\u0019RR>eúQ5uS:N\u001aÿ\n\u0000V\u00000\u0000 \u0000=\u0000 \u0000V\u0000L\u0000*\u0000(\u0000R\u0000O\u0000+\u0000R\u0000L\u0000)\u0000/\u0000R\u0000L\u0000\n\u0000\n\u0000å\rN\t-N\fÿ\u0019RhVöN$Nïz5uS:N\u001aÿ\n\u0000V\u0000L\u0000 \u0000=\u0000 \u0000V\u0000O\u0000*\u0000R\u0000L\u0000/\u0000(\u0000R\u0000O\u0000+\u0000R\u0000L\u0000)\u0000", "V\u0000o\u0000l\u0000t\u0000a\u0000g\u0000e\u0000 \u0000o\u0000n\u0000 \u0000D\u0000U\u0000T\u0000:\u0000 \u0000t\u0000h\u0000e\u0000 \u0000a\u0000c\u0000u\u0000t\u0000a\u0000l\u0000 \u0000v\u0000o\u0000l\u0000t\u0000a\u0000g\u0000e\u0000 \u0000o\u0000n\u0000 \u0000D\u0000U\u0000T\u0000,\u0000 \u0000b\u0000e\u0000c\u0000a\u0000u\u0000s\u0000e\u0000 \u0000t\u0000h\u0000e\u0000 \u0000v\u0000o\u0000l\u0000t\u0000a\u0000g\u0000e\u0000 \u0000o\u0000f\u0000 \u0000A\u0000m\u0000p\u0000 \u0000w\u0000i\u0000l\u0000l\u0000 \u0000b\u0000e\u0000 \u0000d\u0000i\u0000v\u0000i\u0000d\u0000e\u0000d\u0000 \u0000b\u0000y\u0000 \u0000O\u0000u\u0000t\u0000p\u0000u\u0000t\u0000 \u0000I\u0000m\u0000p\u0000e\u0000d\u0000a\u0000n\u0000c\u0000e\u0000\n\u0000A\u0000m\u0000p\u0000 \u0000o\u0000u\u0000t\u0000p\u0000u\u0000t\u0000 \u0000v\u0000o\u0000l\u0000t\u0000a\u0000g\u0000e\u0000\u001aÿV\u0000O\u0000\n\u0000V\u0000o\u0000l\u0000t\u0000a\u0000g\u0000e\u0000 \u0000o\u0000n\u0000 \u0000D\u0000U\u0000T\u0000\u001aÿV\u0000L\u0000\n\u0000O\u0000u\u0000t\u0000p\u0000u\u0000t\u0000 \u0000I\u0000m\u0000p\u0000e\u0000d\u0000a\u0000n\u0000c\u0000e\u0000\u001aÿR\u0000O\u0000\n\u0000N\u0000o\u0000m\u0000i\u0000n\u0000a\u0000l\u0000 \u0000I\u0000m\u0000p\u0000e\u0000d\u0000a\u0000n\u0000c\u0000e\u0000\u001aÿR\u0000L\u0000\n\u0000I\u0000f\u0000 \u0000c\u0000h\u0000e\u0000c\u0000k\u0000 \u0000\"\u0000V\u0000o\u0000l\u0000t\u0000a\u0000g\u0000e\u0000 \u0000o\u0000n\u0000 \u0000D\u0000U\u0000T\u0000\"\u0000 \u0000b\u0000o\u0000x\u0000,\u0000 \u0000t\u0000h\u0000e\u0000 \u0000A\u0000m\u0000p\u0000 \u0000o\u0000u\u0000t\u0000p\u0000u\u0000t\u0000 \u0000v\u0000o\u0000l\u0000t\u0000a\u0000g\u0000e\u0000 \u0000c\u0000a\u0000n\u0000 \u0000b\u0000e\u0000 \u0000c\u0000a\u0000l\u0000c\u0000u\u0000l\u0000a\u0000t\u0000e\u0000d\u0000 \u0000a\u0000s\u0000\u001aÿ\n\u0000V\u00000\u0000 \u0000=\u0000 \u0000V\u0000L\u0000*\u0000(\u0000R\u0000O\u0000+\u0000R\u0000L\u0000)\u0000/\u0000R\u0000L\u0000\n\u0000I\u0000f\u0000 \u0000n\u0000o\u0000t\u0000 \u0000c\u0000h\u0000e\u0000c\u0000k\u0000 \u0000t\u0000h\u0000a\u0000t\u0000 \u0000..."]]  # Tooltip
  # "Voltage on DUT: the acutal voltage on DUT, because the voltage of Amp will be divided by Output Impedance\nAmp output voltageÿVO\nVoltage on DUTÿVL\nOutput ImpedanceÿRO\nNominal ImpedanceÿRL\nIf check \"Voltage on DUT\" box, the Amp output voltage can be calculated asÿ\nV0 = VL*(RO+RL)/RL\nIf not check that box, the Voltage on DUT can be calculated as:\nVL = VO*RL/(RO+RL)"
  # "Caption, Tab Page, Multilist Header, Button 4"
  # "Control Type"
  # "Control Name and Tab"
  n1 = call "CRYSet Front Panel.vi"("Tooltip"=w1, "Caption(Boolean Text)"=string[][] [["S\u0000e\u0000t\u0000t\u0000i\u0000n\u0000g\u0000,\u0000H\u0000e\u0000l\u0000p\u0000", "¾‹n,\u0000.^©R", "$Á\u0015È,\u0000Ä³ÀÆÐ¹"], ["S\u0000t\u0000a\u0000r\u0000t\u0000(\u0000H\u0000z\u0000)\u0000", "\u0000_ËY(\u0000H\u0000z\u0000)\u0000", "ÜÂ‘Ç(\u0000H\u0000z\u0000)\u0000"], ["S\u0000t\u0000o\u0000p\u0000(\u0000H\u0000z\u0000)\u0000", "\\Pbk(\u0000H\u0000z\u0000)\u0000", "\u0015ÈÀÉ(\u0000H\u0000z\u0000)\u0000"], ["R\u0000e\u0000s\u0000o\u0000l\u0000u\u0000t\u0000i\u0000o\u0000n\u0000", "\u0006R¨s", "„½tÕ¥²"], ["S\u0000t\u0000e\u0000p\u0000s\u0000", "ek¤špe", "x¬LÇ"], ["M\u0000i\u0000n\u0000C\u0000y\u0000c\u0000l\u0000e\u0000", "\u0000g\u000f\\hT\u001fgpe", "\\ÍŒÁüÈ0®"], ["M\u0000i\u0000n\u0000 \u0000D\u0000u\u0000r\u0000a\u0000t\u0000i\u0000o\u0000n\u0000(\u0000s\u0000)\u0000", "\u0000gíw\u0001cí~öeô•(\u0000s\u0000)\u0000", "\\ÍŒÁÜÂ\u0004¬(\u0000s\u0000)\u0000"], ["T\u0000r\u0000a\u0000n\u0000s\u0000i\u0000t\u0000i\u0000o\u0000n\u0000", "lbcs", "tÇ‰ÕüÈ\fÓ\u0018Â"], ["U\u0000s\u0000e\u0000M\u0000L\u0000V\u0000a\u0000l\u0000_\u0000L\u0000e\u0000v\u0000e\u0000l\u0000_\u00001\u0000,\u0000S\u0000e\u0000t\u0000 \u0000V\u0000a\u0000l\u0000u\u0000e\u0000,\u0000C\u0000u\u0000r\u0000v\u0000e\u0000s\u0000 \u0000L\u0000i\u0000b\u0000r\u0000a\u0000r\u0000y\u0000(\u0000R\u0000M\u0000S\u0000)\u0000", "O(u<P,\u0000¾‹š[<P,\u0000òf¿~“^", "\u0012¬¬¹©Æ,\u0000\u0012¬$Á\u0015È,\u0000á¬ Á\u001cÁà¬¬¹©Æ"], ["S\u0000t\u0000a\u0000r\u0000t\u0000(\u0000H\u0000z\u0000)\u0000", "\u0000_ËY(\u0000H\u0000z\u0000)\u0000", "ÜÂ‘Ç(\u0000H\u0000z\u0000)\u0000"], ["S\u0000t\u0000o\u0000p\u0000(\u0000H\u0000z\u0000)\u0000", "\\Pbk(\u0000H\u0000z\u0000)\u0000", "\u0015ÈÀÉ(\u0000H\u0000z\u0000)\u0000"], ["S\u0000w\u0000e\u0000e\u0000p\u0000 \u0000R\u0000a\u0000t\u0000e\u0000(\u0000s\u0000/\u0000d\u0000e\u0000c\u0000)\u0000", "kb\u001fs(\u0000s\u0000/\u0000d\u0000e\u0000c\u0000)\u0000", "üÈ¬À`¹(\u0000s\u0000/\u0000d\u0000e\u0000c\u0000)\u0000"], ["U\u0000s\u0000e\u0000M\u0000L\u0000V\u0000a\u0000l\u0000_\u0000L\u0000e\u0000v\u0000e\u0000l\u0000_\u00002\u0000,\u0000S\u0000e\u0000t\u0000 \u0000V\u0000a\u0000l\u0000u\u0000e\u0000,\u0000C\u0000u\u0000r\u0000v\u0000e\u0000s\u0000 \u0000L\u0000i\u0000b\u0000r\u0000a\u0000r\u0000y\u0000(\u0000R\u0000M\u0000S\u0000)\u0000", "O(u<P,\u0000¾‹š[<P,\u0000òf¿~“^", "\u0012¬¬¹©Æ,\u0000\u0012¬$Á\u0015È,\u0000á¬ Á\u001cÁà¬¬¹©Æ"], ["S\u0000t\u0000e\u0000p\u0000s\u0000", "ek¤špe", "x¬LÇ"], ["S\u0000t\u0000a\u0000r\u0000t\u0000", "\u0000_ËY", "ÜÂ‘Ç"], ["S\u0000t\u0000o\u0000p\u0000", "\\Pbk", "\u0015ÈÀÉ"], ["C\u0000y\u0000c\u0000l\u0000e\u0000s\u0000", "hT\u001fg", "üÈ0®"], ["U\u0000s\u0000e\u0000M\u0000L\u0000V\u0000a\u0000l\u0000_\u0000L\u0000e\u0000v\u0000e\u0000l\u0000_\u00003\u0000,\u0000S\u0000e\u0000t\u0000 \u0000V\u0000a\u0000l\u0000u\u0000e\u0000,\u0000C\u0000u\u0000r\u0000v\u0000e\u0000s\u0000 \u0000L\u0000i\u0000b\u0000r\u0000a\u0000r\u0000y\u0000(\u0000R\u0000M\u0000S\u0000)\u0000", "O(u<P,\u0000¾‹š[<P,\u0000òf¿~“^", "\u0012¬¬¹©Æ,\u0000\u0012¬$Á\u0015È,\u0000á¬ Á\u001cÁà¬¬¹©Æ"], ["S\u0000t\u0000e\u0000p\u0000 \u0000S\u0000i\u0000z\u0000e\u0000", "ek•", "x¬LÇlÐ0®"], ["U\u0000s\u0000e\u0000M\u0000L\u0000V\u0000a\u0000l\u0000_\u0000L\u0000e\u0000v\u0000e\u0000l\u0000_\u00004\u0000,\u0000S\u0000e\u0000t\u0000 \u0000V\u0000a\u0000l\u0000u\u0000e\u0000,\u0000C\u0000u\u0000r\u0000v\u0000e\u0000s\u0000 \u0000L\u0000i\u0000b\u0000r\u0000a\u0000r\u0000y\u0000(\u0000R\u0000M\u0000S\u0000)\u0000", "O(u<P,\u0000¾‹š[<P,\u0000òf¿~“^", "\u0012¬¬¹©Æ,\u0000\u0012¬$Á\u0015È,\u0000á¬ Á\u001cÁà¬¬¹©Æ"], ["W\u0000a\u0000v\u0000e\u0000 \u0000F\u0000i\u0000l\u0000e\u0000 \u0000P\u0000a\u0000t\u0000h\u0000", "âlb_eöNï_", "ÜÂ\u0004¬\fÓ\u0015Ö\fÓ|Ç½¬\\¸"], ["R\u0000M\u0000S\u0000", "R\u0000M\u0000S\u0000", "R\u0000M\u0000S\u0000"], ["P\u0000e\u0000a\u0000k\u0000", "ð\\<P", "\\Í\u0000³\u0012¬"], ["C\u0000o\u0000n\u0000t\u0000r\u0000o\u0000l\u0000 \u0000M\u0000e\u0000t\u0000h\u0000o\u0000d\u0000,\u0000U\u0000S\u0000B\u0000,\u0000a\u0000n\u0000a\u0000l\u0000o\u0000g\u0000", "§c6R¹eÕl,\u0000U\u0000S\u0000B\u0000,\u0000!jßb", "pÈ…È)¼•¼,\u0000U\u0000S\u0000B\u0000,\u0000ÁÀ¬À"], ["S\u0000o\u0000u\u0000r\u0000c\u0000e\u0000 \u0000T\u0000y\u0000p\u0000e\u0000,\u0000v\u0000o\u0000l\u0000t\u0000a\u0000g\u0000e\u0000,\u0000c\u0000u\u0000r\u0000r\u0000e\u0000n\u0000t\u0000", "n{|W,\u00005uS,\u00005uAm", "ÐÆœÌ\u0015ÖÜÐ,\u0000\u0004ÈUÅ,\u0000\u0004ÈX¹"], ["P\u0000o\u0000l\u0000a\u0000r\u0000i\u0000t\u0000y\u0000,\u0000p\u0000o\u0000s\u0000i\u0000t\u0000i\u0000v\u0000e\u0000,\u0000n\u0000e\u0000g\u0000a\u0000t\u0000i\u0000v\u0000e\u0000", "g'`,\u0000ck,\u0000\u001f", "ù­1Á,\u0000\u0015È,\u0000€½"], ["M\u0000a\u0000x\u0000.\u0000C\u0000u\u0000r\u0000r\u0000e\u0000n\u0000t\u0000", "\u0000g'Y5uAm", "\\Í\u0000³\u0004ÈX¹"], ["S\u0000t\u0000e\u0000p\u0000s\u0000", "ek¤špe", "x¬LÇ"], ["T\u0000i\u0000m\u0000e\u0000/\u0000S\u0000t\u0000e\u0000p\u0000(\u0000s\u0000)\u0000", "öeô•/\u0000ek(\u0000s\u0000)\u0000", "ÜÂ\u0004¬/\u0000x¬LÇ(\u0000s\u0000)\u0000"], ["S\u0000t\u0000a\u0000r\u0000t\u0000", "\u0000_ËY", "ÜÂ‘Ç"], ["S\u0000t\u0000o\u0000p\u0000", "\\Pbk", "\u0015ÈÀÉ"], ["L\u0000e\u0000v\u0000e\u0000l\u0000", "E^¦^", "\u0000É\u0004Ç"], ["S\u0000t\u0000e\u0000p\u0000s\u0000 \u0000S\u0000i\u0000z\u0000e\u0000", "ek•", "x¬LÇlÐ0®"], ["S\u0000w\u0000e\u0000e\u0000p\u0000 \u0000T\u0000y\u0000p\u0000e\u0000,\u0000I\u0000M\u0000,\u0000D\u0000i\u0000f\u0000f\u0000e\u0000r\u0000e\u0000n\u0000c\u0000e\u0000", "kbÏc{|‹W,\u0000’N\u0003ŒáO÷S,\u0000î]‘˜áO÷S", "üÈ¬À\u0015ÖÜÐ,\u00008ÖÁÀÀ¼pÈ,\u0000(ÌtÇ"], ["S\u0000t\u0000a\u0000r\u0000t\u0000(\u0000H\u0000z\u0000)\u0000", "\u0000_ËY(\u0000H\u0000z\u0000)\u0000", "ÜÂ‘Ç(\u0000H\u0000z\u0000)\u0000"], ["S\u0000t\u0000o\u0000p\u0000(\u0000H\u0000z\u0000)\u0000", "\\Pbk(\u0000H\u0000z\u0000)\u0000", "\u0015ÈÀÉ(\u0000H\u0000z\u0000)\u0000"], ["U\u0000s\u0000e\u0000M\u0000L\u0000V\u0000a\u0000l\u0000_\u0000L\u0000e\u0000v\u0000e\u0000l\u00006\u0000_\u00001\u0000,\u0000S\u0000e\u0000t\u0000 \u0000V\u0000a\u0000l\u0000u\u0000e\u0000,\u0000C\u0000u\u0000r\u0000v\u0000e\u0000s\u0000 \u0000L\u0000i\u0000b\u0000r\u0000a\u0000r\u0000y\u0000(\u0000R\u0000M\u0000S\u0000)\u0000", "O(u<P,\u0000¾‹š[<P,\u0000òf¿~“^", "\u0012¬¬¹©Æ,\u0000\u0012¬$Á\u0015È,\u0000á¬ Á\u001cÁà¬¬¹©Æ"], ["F\u0000i\u0000x\u0000e\u0000d\u0000/\u0000R\u0000a\u0000t\u0000i\u0000o\u00006\u0000,\u0000F\u0000i\u0000x\u0000e\u0000d\u0000,\u0000R\u0000a\u0000t\u0000i\u0000o\u0000", "úVš[/\u0000Ôk‡s,\u0000úVš[,\u0000Ôk‡s", "à¬\u0015È/\u0000D¾`¹,\u0000à¬\u0015È,\u0000D¾`¹"], ["U\u0000s\u0000e\u0000M\u0000L\u0000V\u0000a\u0000l\u0000_\u0000L\u0000e\u0000v\u0000e\u0000l\u00006\u0000_\u00002\u0000,\u0000S\u0000e\u0000t\u0000 \u0000V\u0000a\u0000l\u0000u\u0000e\u0000,\u0000C\u0000u\u0000r\u0000v\u0000e\u0000s\u0000 \u0000L\u0000i\u0000b\u0000r\u0000a\u0000r\u0000y\u0000(\u0000R\u0000M\u0000S\u0000)\u0000", "O(u<P,\u0000¾‹š[<P,\u0000òf¿~“^", "\u0012¬¬¹©Æ,\u0000\u0012¬$Á\u0015È,\u0000á¬ Á\u001cÁà¬¬¹©Æ"], ["T\u0000r\u0000a\u0000n\u0000s\u0000i\u0000t\u0000i\u0000o\u0000n\u0000", "lbcs", "tÇ‰ÕüÈ\fÓ\u0018Â"], ["R\u0000e\u0000s\u0000o\u0000l\u0000u\u0000t\u0000i\u0000o\u0000n\u0000", "\u0006R¨s", "„½tÕ¥²"], ["S\u0000t\u0000e\u0000p\u0000s\u0000", "ek¤špe", "x¬LÇ"], ["M\u0000i\u0000n\u0000 \u0000C\u0000y\u0000c\u0000l\u0000e\u0000", "\u0000g\u000f\\hT\u001fgpe", "\\ÍŒÁüÈ0®"], ["M\u0000i\u0000n\u0000 \u0000D\u0000u\u0000r\u0000a\u0000t\u0000i\u0000o\u0000n\u0000(\u0000s\u0000)\u0000", "\u0000gíw\u0001cí~öeô•(\u0000s\u0000)\u0000", "\\ÍŒÁÜÂ\u0004¬(\u0000s\u0000)\u0000"], ["D\u0000i\u0000f\u0000f\u0000e\u0000r\u0000e\u0000n\u0000c\u0000e\u0000(\u0000H\u0000z\u0000)\u0000", "î]\u0002_(\u0000H\u0000z\u0000)\u0000", "(ÌtÇ(\u0000H\u0000z\u0000)\u0000"], ["R\u0000a\u0000t\u0000i\u0000o\u0000", "Ôk‡s", "D¾`¹"], ["M\u0000a\u0000s\u0000t\u0000e\u0000r\u0000 \u0000T\u0000o\u0000n\u0000e\u0000,\u0000S\u0000l\u0000a\u0000v\u0000e\u0000 \u0000T\u0000o\u0000n\u0000e\u0000", ";Nó—áO÷S,\u0000ÎNó—áO÷S", "0®ø¼LÇ,\u0000ô¼pÈLÇ"], ["N\u0000o\u0000i\u0000s\u0000e\u0000 \u0000T\u0000y\u0000p\u0000e\u00007\u0000,\u0000P\u0000i\u0000n\u0000k\u0000 \u0000N\u0000o\u0000i\u0000s\u0000e\u0000,\u0000W\u0000h\u0000i\u0000t\u0000e\u0000 \u0000N\u0000o\u0000i\u0000s\u0000e\u0000", "jVðX{|‹W,\u0000‰|¢~jVðX,\u0000}vjVðX", "¡ÇLÇ\u0015ÖÜÐ,\u0000„½MÖÉÀ¡ÇLÇ,\u00001¼ÉÀ¡ÇLÇ"], ["D\u0000u\u0000r\u0000a\u0000t\u0000i\u0000o\u0000n\u0000(\u0000s\u0000)\u0000", "öeô•(\u0000s\u0000)\u0000", "ÀÉÁÜÂ\u0004¬(\u0000s\u0000)\u0000"], ["S\u0000t\u0000a\u0000r\u0000t\u0000(\u0000H\u0000z\u0000)\u0000", "\u0000_ËY(\u0000H\u0000z\u0000)\u0000", "ÜÂ‘Ç(\u0000H\u0000z\u0000)\u0000"], ["S\u0000t\u0000o\u0000p\u0000(\u0000H\u0000z\u0000)\u0000", "\\Pbk(\u0000H\u0000z\u0000)\u0000", "\u0015ÈÀÉ(\u0000H\u0000z\u0000)\u0000"], ["S\u0000t\u0000a\u0000r\u0000t\u0000(\u0000H\u0000z\u0000)\u0000", "\u0000_ËY(\u0000H\u0000z\u0000)\u0000", "ÜÂ‘Ç(\u0000H\u0000z\u0000)\u0000"], ["S\u0000t\u0000o\u0000p\u0000(\u0000H\u0000z\u0000)\u0000", "\\Pbk(\u0000H\u0000z\u0000)\u0000", "\u0015ÈÀÉ(\u0000H\u0000z\u0000)\u0000"], ["U\u0000s\u0000e\u0000M\u0000L\u0000V\u0000a\u0000l\u0000_\u0000L\u0000e\u0000v\u0000e\u0000l\u0000_\u00007\u0000,\u0000S\u0000e\u0000t\u0000 \u0000V\u0000a\u0000l\u0000u\u0000e\u0000,\u0000C\u0000u\u0000r\u0000v\u0000e\u0000s\u0000 \u0000L\u0000i\u0000b\u0000r\u0000a\u0000r\u0000y\u0000(\u0000R\u0000M\u0000S\u0000)\u0000", "O(u<P,\u0000¾‹š[<P,\u0000òf¿~“^", "\u0012¬¬¹©Æ,\u0000\u0012¬$Á\u0015È,\u0000á¬ Á\u001cÁà¬¬¹©Æ"], ["R\u0000e\u0000s\u0000o\u0000l\u0000u\u0000t\u0000i\u0000o\u0000n\u0000", "\u0006R¨s", "„½tÕ¥²"], ["U\u0000s\u0000e\u0000M\u0000L\u0000V\u0000a\u0000l\u0000_\u0000L\u0000e\u0000v\u0000e\u0000l\u0000_\u00008\u0000,\u0000S\u0000e\u0000t\u0000 \u0000V\u0000a\u0000l\u0000u\u0000e\u0000,\u0000C\u0000u\u0000r\u0000v\u0000e\u0000s\u0000 \u0000L\u0000i\u0000b\u0000r\u0000a\u0000r\u0000y\u0000(\u0000R\u0000M\u0000S\u0000)\u0000", "O(u<P,\u0000¾‹š[<P,\u0000òf¿~“^", "\u0012¬¬¹©Æ,\u0000\u0012¬$Á\u0015È,\u0000á¬ Á\u001cÁà¬¬¹©Æ"], ["F\u0000r\u0000e\u0000q\u0000u\u0000e\u0000n\u0000c\u0000y\u0000 \u0000R\u0000o\u0000u\u0000n\u0000d\u0000i\u0000n\u0000g\u0000", "‘˜‡sÛV\r‚”NeQ", "üÈ\fÓ\u0018Âe´ø­¬¹0®"], ["D\u0000u\u0000r\u0000a\u0000t\u0000i\u0000o\u0000n\u0000(\u0000s\u0000)\u0000", "\u0001cí~öeô•(\u0000s\u0000)\u0000", "ÀÉÁÜÂ\u0004¬(\u0000s\u0000)\u0000"], ["T\u0000o\u0000n\u0000e\u0000s\u0000", "\u001aYó—peÏ‘", "LÇpÈ"], ["R\u0000o\u0000u\u0000n\u0000d\u0000i\u0000n\u0000g\u0000 \u0000V\u0000a\u0000l\u0000u\u0000e\u0000(\u0000H\u0000z\u0000)\u0000", "\r‚eQ<P(\u0000H\u0000z\u0000)\u0000", "e´ø­¬¹0®\u0012¬(\u0000H\u0000z\u0000)\u0000"], ["L\u0000e\u0000v\u0000e\u0000l\u0000", "E^¦^", "\u0000É\u0004Ç"], ["S\u0000t\u0000e\u0000p\u0000 \u0000P\u0000r\u0000o\u0000g\u0000r\u0000e\u0000s\u0000s\u0000i\u0000o\u0000n\u0000", "ekÛ¾n", "x¬LÇ$Á\u0015È"], ["F\u0000r\u0000e\u0000q\u0000u\u0000e\u0000n\u0000c\u0000y\u0000 \u0000R\u0000a\u0000n\u0000g\u0000e\u0000", "‘˜‡s\u0003ƒôV", "üÈ\fÓ\u0018Â”¼\u0004Ç"], ["S\u0000t\u0000e\u0000p\u0000 \u0000S\u0000i\u0000z\u0000e\u0000", "ek•", "x¬LÇlÐ0®"], ["L\u0000e\u0000v\u0000e\u0000l\u0000", "E^¦^", "\u0000É\u0004Ç"], ["S\u0000t\u0000e\u0000p\u0000 \u0000P\u0000r\u0000o\u0000g\u0000r\u0000e\u0000s\u0000s\u0000i\u0000o\u0000n\u0000", "ekÛ¾n", "x¬LÇ$Á\u0015È"], ["F\u0000r\u0000e\u0000q\u0000u\u0000e\u0000n\u0000c\u0000y\u0000 \u0000R\u0000a\u0000n\u0000g\u0000e\u0000", "‘˜‡s\u0003ƒôV", "üÈ\fÓ\u0018Â”¼\u0004Ç"], ["F\u0000r\u0000e\u0000q\u0000u\u0000e\u0000n\u0000c\u0000y\u0000(\u0000H\u0000z\u0000)\u0000", "‘˜‡s(\u0000H\u0000z\u0000)\u0000", "üÈ\fÓ\u0018Â(\u0000H\u0000z\u0000)\u0000"], ["S\u0000t\u0000e\u0000p\u0000 \u0000P\u0000r\u0000o\u0000g\u0000r\u0000e\u0000s\u0000s\u0000i\u0000o\u0000n\u0000", "ekÛ¾n", "x¬LÇ$Á\u0015È"], ["L\u0000e\u0000v\u0000e\u0000l\u0000 \u0000R\u0000a\u0000n\u0000g\u0000e\u0000", "E^¦^\u0003ƒôV", "\u0000É\u0004Ç”¼\u0004Ç"], ["W\u0000A\u0000V\u0000 \u0000I\u0000n\u0000f\u0000o\u0000", "W\u0000A\u0000V\u0000áOo`", "ÜÂ\u0004¬\fÓ\u0015Ö\u0015Èô¼"], ["L\u0000e\u0000v\u0000e\u0000l\u0000", "E^¦^", "\u0000É\u0004Ç"], ["I\u0000n\u0000s\u0000t\u0000r\u0000u\u0000m\u0000e\u0000n\u0000t\u0000 \u0000S\u0000e\u0000t\u0000t\u0000i\u0000n\u0000g\u0000s\u0000", "êNhV¾‹n", "Ä¬0®$Á\u0015È"], ["S\u0000w\u0000e\u0000e\u0000p\u0000 \u0000S\u0000e\u0000t\u0000t\u0000i\u0000n\u0000g\u0000s\u0000", "kbÏc¾‹n", "üÈ¬À$Á\u0015È"], ["L\u0000e\u0000v\u0000e\u0000l\u0000 \u0000R\u0000a\u0000n\u0000g\u0000e\u0000", "E^¦^\u0003ƒôV", "\u0000É\u0004Ç”¼\u0004Ç"], ["S\u0000w\u0000e\u0000e\u0000p\u0000 \u0000T\u0000y\u0000p\u0000e\u0000", "kb‘˜{|‹W", "üÈ¬À\u0015ÖÜÐ"], ["L\u0000e\u0000v\u0000e\u0000l\u0000", "E^¦^", "\u0000É\u0004Ç"], ["F\u0000r\u0000e\u0000q\u0000u\u0000e\u0000n\u0000c\u0000y\u0000 \u0000R\u0000a\u0000n\u0000g\u0000e\u0000", "‘˜‡s\u0003ƒôV", "üÈ\fÓ\u0018Â”¼\u0004Ç"], ["S\u0000t\u0000e\u0000p\u0000 \u0000S\u0000i\u0000z\u0000e\u0000", "ek•", "x¬LÇlÐ0®"], ["L\u0000e\u0000v\u0000e\u0000l\u0000", "E^¦^", "\u0000É\u0004Ç"], ["F\u0000i\u0000x\u0000e\u0000d\u0000 \u0000T\u0000o\u0000n\u0000e\u0000(\u0000H\u0000z\u0000)\u0000", "úVš[ó—\u0003Œ(\u0000H\u0000z\u0000)\u0000", "à¬\u0015ÈLÇ(\u0000H\u0000z\u0000)\u0000"], ["L\u0000e\u0000v\u0000e\u0000l\u0000", "E^¦^", "\u0000É\u0004Ç"], ["N\u0000o\u0000i\u0000s\u0000e\u0000", "jVó—", "¡ÇLÇ"], ["F\u0000r\u0000e\u0000q\u0000u\u0000e\u0000n\u0000c\u0000y\u0000 \u0000R\u0000a\u0000n\u0000g\u0000e\u0000", "‘˜‡s\u0003ƒôV", "üÈ\fÓ\u0018Â”¼\u0004Ç"], ["L\u0000e\u0000v\u0000e\u0000l\u0000", "E^¦^", "\u0000É\u0004Ç"], ["M\u0000u\u0000l\u0000t\u0000i\u0000t\u0000o\u0000n\u0000e\u0000", "\u001aY‘˜ó—", "ä²\u0011ÉLÇ"], ["F\u0000r\u0000e\u0000q\u0000u\u0000e\u0000n\u0000c\u0000y\u0000 \u0000R\u0000a\u0000n\u0000g\u0000e\u0000", "‘˜‡s\u0003ƒôV", "üÈ\fÓ\u0018Â”¼\u0004Ç"], ["S\u0000t\u0000i\u0000m\u0000u\u0000l\u0000u\u0000s\u0000 \u0000T\u0000y\u0000p\u0000e\u0000,\u0000F\u0000r\u0000e\u0000q\u0000u\u0000e\u0000n\u0000c\u0000y\u0000 \u0000S\u0000t\u0000e\u0000p\u0000p\u0000e\u0000d\u0000 \u0000S\u0000w\u0000e\u0000e\u0000p\u0000,\u0000F\u0000r\u0000e\u0000q\u0000u\u0000e\u0000n\u0000c\u0000y\u0000 \u0000L\u0000o\u0000g\u0000 \u0000S\u0000w\u0000e\u0000e\u0000p\u0000,\u0000L\u0000o\u0000g\u0000 \u0000A\u0000m\u0000p\u0000l\u0000i\u0000t\u0000u\u0000d\u0000e\u0000 \u0000S\u0000w\u0000e\u0000e\u0000p\u0000,\u0000W\u0000A\u0000V\u0000,\u0000T\u0000w\u0000o\u0000 \u0000T\u0000o\u0000n\u0000e\u0000,\u0000N\u0000o\u0000i\u0000s\u0000e\u0000,\u0000M\u0000u\u0000l\u0000t\u0000i\u0000t\u0000o\u0000n\u0000e\u0000", "Ào±R{|W,\u0000sekÛkb,\u0000sù[pekb,\u0000E^¦^ù[pekb,\u0000W\u0000A\u0000V\u0000eöN,\u0000ÌSóáO÷S,\u0000jVðXáO÷S,\u0000\u001aYóáO÷S", "Çù­àÂ8Ö\u0015ÖÜÐ,\u0000üÈ\fÓ\u0018Âx¬LÇüÈ¬À,\u0000üÈ\fÓ\u0018Â\\¸ø­üÈ¬À,\u0000\\¸ø­ÄÉíÓüÈ¬À,\u0000LÇ1Á\fÓ|Ç,\u0000\rÃLÇpÈàÂ8Ö,\u0000¡ÇLÇàÂ8Ö,\u0000ä²üÈ\fÓàÂ8Ö"], ["O\u0000K\u0000", "nxš[", "UÖxÇ"], ["C\u0000a\u0000n\u0000c\u0000e\u0000l\u0000", "ÖSˆm", "èÍŒÁ"], ["C\u0000h\u0000a\u0000n\u0000n\u0000e\u0000l\u0000", "\u001aS", "µÑ\\¸"], ["M\u0000e\u0000s\u0000s\u0000a\u0000g\u0000e\u0000,\u0000S\u0000t\u0000a\u0000r\u0000t\u0000(\u0000H\u0000z\u0000)\u0000", "M\u0000e\u0000s\u0000s\u0000a\u0000g\u0000e\u0000,\u0000\u0000_ËY(\u0000H\u0000z\u0000)\u0000", "M\u0000e\u0000s\u0000s\u0000a\u0000g\u0000e\u0000,\u0000ÜÂ‘Ç(\u0000H\u0000z\u0000)\u0000"], ["M\u0000e\u0000s\u0000s\u0000a\u0000g\u0000e\u0000,\u0000S\u0000t\u0000o\u0000p\u0000(\u0000H\u0000z\u0000)\u0000", "M\u0000e\u0000s\u0000s\u0000a\u0000g\u0000e\u0000,\u0000\\Pbk(\u0000H\u0000z\u0000)\u0000", "M\u0000e\u0000s\u0000s\u0000a\u0000g\u0000e\u0000,\u0000\u0015ÈÀÉ(\u0000H\u0000z\u0000)\u0000"], ["M\u0000e\u0000s\u0000s\u0000a\u0000g\u0000e\u0000,\u0000S\u0000t\u0000a\u0000r\u0000t\u0000(\u0000H\u0000z\u0000)\u0000", "M\u0000e\u0000s\u0000s\u0000a\u0000g\u0000e\u0000,\u0000\u0000_ËY(\u0000H\u0000z\u0000)\u0000", "M\u0000e\u0000s\u0000s\u0000a\u0000g\u0000e\u0000,\u0000ÜÂ‘Ç(\u0000H\u0000z\u0000)\u0000"], ["M\u0000e\u0000s\u0000s\u0000a\u0000g\u0000e\u0000,\u0000S\u0000t\u0000o\u0000p\u0000(\u0000H\u0000z\u0000)\u0000", "M\u0000e\u0000s\u0000s\u0000a\u0000g\u0000e\u0000,\u0000\\Pbk(\u0000H\u0000z\u0000)\u0000", "M\u0000e\u0000s\u0000s\u0000a\u0000g\u0000e\u0000,\u0000\u0015ÈÀÉ(\u0000H\u0000z\u0000)\u0000"], ["M\u0000e\u0000s\u0000s\u0000a\u0000g\u0000e\u0000,\u0000S\u0000t\u0000a\u0000r\u0000t\u0000(\u0000H\u0000z\u0000)\u0000", "M\u0000e\u0000s\u0000s\u0000a\u0000g\u0000e\u0000,\u0000\u0000_ËY(\u0000H\u0000z\u0000)\u0000", "M\u0000e\u0000s\u0000s\u0000a\u0000g\u0000e\u0000,\u0000ÜÂ‘Ç(\u0000H\u0000z\u0000)\u0000"], ["M\u0000e\u0000s\u0000s\u0000a\u0000g\u0000e\u0000,\u0000S\u0000t\u0000o\u0000p\u0000(\u0000H\u0000z\u0000)\u0000", "M\u0000e\u0000s\u0000s\u0000a\u0000g\u0000e\u0000,\u0000\\Pbk(\u0000H\u0000z\u0000)\u0000", "M\u0000e\u0000s\u0000s\u0000a\u0000g\u0000e\u0000,\u0000\u0015ÈÀÉ(\u0000H\u0000z\u0000)\u0000"], ["M\u0000e\u0000s\u0000s\u0000a\u0000g\u0000e\u0000,\u0000S\u0000t\u0000a\u0000r\u0000t\u0000(\u0000H\u0000z\u0000)\u0000", "M\u0000e\u0000s\u0000s\u0000a\u0000g\u0000e\u0000,\u0000\u0000_ËY(\u0000H\u0000z\u0000)\u0000", "M\u0000e\u0000s\u0000s\u0000a\u0000g\u0000e\u0000,\u0000ÜÂ‘Ç(\u0000H\u0000z\u0000)\u0000"], ["M\u0000e\u0000s\u0000s\u0000a\u0000g\u0000e\u0000,\u0000S\u0000t\u0000o\u0000p\u0000(\u0000H\u0000z\u0000)\u0000", "M\u0000e\u0000s\u0000s\u0000a\u0000g\u0000e\u0000,\u0000\\Pbk(\u0000H\u0000z\u0000)\u0000", "M\u0000e\u0000s\u0000s\u0000a\u0000g\u0000e\u0000,\u0000\u0015ÈÀÉ(\u0000H\u0000z\u0000)\u0000"], ["M\u0000e\u0000s\u0000s\u0000a\u0000g\u0000e\u0000,\u0000S\u0000t\u0000a\u0000r\u0000t\u0000(\u0000H\u0000z\u0000)\u0000", "M\u0000e\u0000s\u0000s\u0000a\u0000g\u0000e\u0000,\u0000\u0000_ËY(\u0000H\u0000z\u0000)\u0000", "M\u0000e\u0000s\u0000s\u0000a\u0000g\u0000e\u0000,\u0000ÜÂ‘Ç(\u0000H\u0000z\u0000)\u0000"], ["M\u0000e\u0000s\u0000s\u0000a\u0000g\u0000e\u0000,\u0000S\u0000t\u0000o\u0000p\u0000(\u0000H\u0000z\u0000)\u0000", "M\u0000e\u0000s\u0000s\u0000a\u0000g\u0000e\u0000,\u0000\\Pbk(\u0000H\u0000z\u0000)\u0000", "M\u0000e\u0000s\u0000s\u0000a\u0000g\u0000e\u0000,\u0000\u0015ÈÀÉ(\u0000H\u0000z\u0000)\u0000"], ["O\u0000u\u0000t\u0000p\u0000u\u0000t\u0000 \u0000I\u0000m\u0000p\u0000.\u0000,\u00001\u0000,\u00003\u00003\u0000,\u00001\u00005\u00000\u0000,\u00006\u00000\u00000\u0000,\u00007\u00005\u00000\u0000", "úQ;b,\u00001\u0000,\u00003\u00003\u0000,\u00001\u00005\u00000\u0000,\u00006\u00000\u00000\u0000,\u00007\u00005\u00000\u0000", "O\u0000u\u0000t\u0000p\u0000u\u0000t\u0000 \u0000I\u0000m\u0000p\u0000.\u0000,\u00001\u0000,\u00003\u00003\u0000,\u00001\u00005\u00000\u0000,\u00006\u00000\u00000\u0000,\u00007\u00005\u00000\u0000"], ["N\u0000o\u0000m\u0000i\u0000n\u0000a\u0000l\u0000 \u0000I\u0000m\u0000p\u0000.\u0000", "[;b", "N\u0000o\u0000m\u0000i\u0000n\u0000a\u0000l\u0000 \u0000I\u0000m\u0000p\u0000.\u0000"], ["V\u0000o\u0000l\u0000t\u0000a\u0000g\u0000e\u0000 \u0000o\u0000n\u0000 \u0000D\u0000U\u0000T\u0000(\u0000?\u0000)\u0000", "hVöN$Nïz5u‹S(\u0000?\u0000)\u0000", "V\u0000o\u0000l\u0000t\u0000a\u0000g\u0000e\u0000 \u0000o\u0000n\u0000 \u0000D\u0000U\u0000T\u0000(\u0000?\u0000)\u0000"], ["O\u0000u\u0000t\u0000p\u0000u\u0000t\u0000 \u0000I\u0000m\u0000p\u0000.\u0000,\u00001\u0000,\u00003\u00003\u0000,\u00001\u00005\u00000\u0000,\u00006\u00000\u00000\u0000,\u00007\u00005\u00000\u0000", "úQ;b,\u00001\u0000,\u00003\u00003\u0000,\u00001\u00005\u00000\u0000,\u00006\u00000\u00000\u0000,\u00007\u00005\u00000\u0000", "O\u0000u\u0000t\u0000p\u0000u\u0000t\u0000 \u0000I\u0000m\u0000p\u0000.\u0000,\u00001\u0000,\u00003\u00003\u0000,\u00001\u00005\u00000\u0000,\u00006\u00000\u00000\u0000,\u00007\u00005\u00000\u0000"], ["N\u0000o\u0000m\u0000i\u0000n\u0000a\u0000l\u0000 \u0000I\u0000m\u0000p\u0000.\u0000", "[;b", "N\u0000o\u0000m\u0000i\u0000n\u0000a\u0000l\u0000 \u0000I\u0000m\u0000p\u0000.\u0000"], ["V\u0000o\u0000l\u0000t\u0000a\u0000g\u0000e\u0000 \u0000o\u0000n\u0000 \u0000D\u0000U\u0000T\u0000(\u0000?\u0000)\u0000", "hVöN$Nïz5u‹S(\u0000?\u0000)\u0000", "V\u0000o\u0000l\u0000t\u0000a\u0000g\u0000e\u0000 \u0000o\u0000n\u0000 \u0000D\u0000U\u0000T\u0000(\u0000?\u0000)\u0000"], ["O\u0000u\u0000t\u0000p\u0000u\u0000t\u0000 \u0000I\u0000m\u0000p\u0000.\u0000,\u00001\u0000,\u00003\u00003\u0000,\u00001\u00005\u00000\u0000,\u00006\u00000\u00000\u0000,\u00007\u00005\u00000\u0000", "úQ;b,\u00001\u0000,\u00003\u00003\u0000,\u00001\u00005\u00000\u0000,\u00006\u00000\u00000\u0000,\u00007\u00005\u00000\u0000", "O\u0000u\u0000t\u0000p\u0000u\u0000t\u0000 \u0000I\u0000m\u0000p\u0000.\u0000,\u00001\u0000,\u00003\u00003\u0000,\u00001\u00005\u00000\u0000,\u00006\u00000\u00000\u0000,\u00007\u00005\u00000\u0000"], ["N\u0000o\u0000m\u0000i\u0000n\u0000a\u0000l\u0000 \u0000I\u0000m\u0000p\u0000.\u0000", "[;b", "N\u0000o\u0000m\u0000i\u0000n\u0000a\u0000l\u0000 \u0000I\u0000m\u0000p\u0000.\u0000"], ["V\u0000o\u0000l\u0000t\u0000a\u0000g\u0000e\u0000 \u0000o\u0000n\u0000 \u0000D\u0000U\u0000T\u0000(\u0000?\u0000)\u0000", "hVöN$Nïz5u‹S(\u0000?\u0000)\u0000", "V\u0000o\u0000l\u0000t\u0000a\u0000g\u0000e\u0000 \u0000o\u0000n\u0000 \u0000D\u0000U\u0000T\u0000(\u0000?\u0000)\u0000"], ["O\u0000u\u0000t\u0000p\u0000u\u0000t\u0000 \u0000I\u0000m\u0000p\u0000.\u0000,\u00001\u0000,\u00003\u00003\u0000,\u00001\u00005\u00000\u0000,\u00006\u00000\u00000\u0000,\u00007\u00005\u00000\u0000", "úQ;b,\u00001\u0000,\u00003\u00003\u0000,\u00001\u00005\u00000\u0000,\u00006\u00000\u00000\u0000,\u00007\u00005\u00000\u0000", "O\u0000u\u0000t\u0000p\u0000u\u0000t\u0000 \u0000I\u0000m\u0000p\u0000.\u0000,\u00001\u0000,\u00003\u00003\u0000,\u00001\u00005\u00000\u0000,\u00006\u00000\u00000\u0000,\u00007\u00005\u00000\u0000"], ["N\u0000o\u0000m\u0000i\u0000n\u0000a\u0000l\u0000 \u0000I\u0000m\u0000p\u0000.\u0000", "[;b", "N\u0000o\u0000m\u0000i\u0000n\u0000a\u0000l\u0000 \u0000I\u0000m\u0000p\u0000.\u0000"], ["V\u0000o\u0000l\u0000t\u0000a\u0000g\u0000e\u0000 \u0000o\u0000n\u0000 \u0000D\u0000U\u0000T\u0000(\u0000?\u0000)\u0000", "hVöN$Nïz5u‹S(\u0000?\u0000)\u0000", "V\u0000o\u0000l\u0000t\u0000a\u0000g\u0000e\u0000 \u0000o\u0000n\u0000 \u0000D\u0000U\u0000T\u0000(\u0000?\u0000)\u0000"], ["O\u0000u\u0000t\u0000p\u0000u\u0000t\u0000 \u0000I\u0000m\u0000p\u0000.\u0000,\u00001\u0000,\u00003\u00003\u0000,\u00001\u00005\u00000\u0000,\u00006\u00000\u00000\u0000,\u00007\u00005\u00000\u0000", "úQ;b,\u00001\u0000,\u00003\u00003\u0000,\u00001\u00005\u00000\u0000,\u00006\u00000\u00000\u0000,\u00007\u00005\u00000\u0000", "O\u0000u\u0000t\u0000p\u0000u\u0000t\u0000 \u0000I\u0000m\u0000p\u0000.\u0000,\u00001\u0000,\u00003\u00003\u0000,\u00001\u00005\u00000\u0000,\u00006\u00000\u00000\u0000,\u00007\u00005\u00000\u0000"], ["N\u0000o\u0000m\u0000i\u0000n\u0000a\u0000l\u0000 \u0000I\u0000m\u0000p\u0000.\u0000", "[;b", "N\u0000o\u0000m\u0000i\u0000n\u0000a\u0000l\u0000 \u0000I\u0000m\u0000p\u0000.\u0000"], ["V\u0000o\u0000l\u0000t\u0000a\u0000g\u0000e\u0000 \u0000o\u0000n\u0000 \u0000D\u0000U\u0000T\u0000(\u0000?\u0000)\u0000", "hVöN$Nïz5u‹S(\u0000?\u0000)\u0000", "V\u0000o\u0000l\u0000t\u0000a\u0000g\u0000e\u0000 \u0000o\u0000n\u0000 \u0000D\u0000U\u0000T\u0000(\u0000?\u0000)\u0000"]], "Control ID and Type(Label Name, Type)"=string[][] [["Board1 Tab", "Tab"], ["StartFreq1(Hz)", "Numeric"], ["StopFreq1(Hz)", "Numeric"], ["Step Resolution1", "Ring"], ["Steps1", "Numeric"], ["Cycle/step1", "Numeric"], ["Time/steps1(s)", "Numeric"], ["Transition1", "Numeric"], ["UseMLVal_Level_1", "Slide"], ["StartFreq2(Hz)", "Numeric"], ["StopFreq2(Hz)", "Numeric"], ["Sweept Rate2(s/dec)", "Numeric"], ["UseMLVal_Level_2", "Slide"], ["Steps3", "Numeric"], ["Start Amp3", "Numeric"], ["Stop Amp3", "Numeric"], ["Cycles3", "Numeric"], ["UseMLVal_Level_3", "Slide"], ["Step Size3", "Numeric"], ["UseMLVal_Level_4", "Slide"], ["Wave Path4", "Path"], ["RMS value4", "Numeric"], ["Peak value4", "Numeric"], ["dc_ctrl5_1", "Slide"], ["dc_ctrl5_2", "Slide"], ["dcpolar5", "Slide"], ["Max.Current", "Slide"], ["Steps5", "Numeric"], ["Time/Step5", "Numeric"], ["StartAmp5", "Numeric"], ["StopAmp5", "Numeric"], ["Level5", "Numeric"], ["Steps Size5", "Numeric"], ["Sweep Type", "Slide"], ["StartFreq6(Hz)", "Numeric"], ["StopFreq6(Hz)", "Numeric"], ["UseMLVal_Level6_1", "Slide"], ["Fixed/Ratio6", "Slide"], ["UseMLVal_Level6_2", "Slide"], ["Transition6", "Numeric"], ["StepResolution6", "Ring"], ["Steps6", "Numeric"], ["Cycle/steps6", "Numeric"], ["Time/step6(s)", "Numeric"], ["Difference6(Hz)", "Numeric"], ["Ratio6", "Ring"], ["Control6 Tab", "Tab"], ["Noise Type7", "Slide"], ["Duration7(s)", "Numeric"], ["Min Freq7(Hz)", "Numeric"], ["Max Freq7(Hz)", "Numeric"], ["Min Freq8(Hz)", "Numeric"], ["Max Freq8(Hz)", "Numeric"], ["UseMLVal_Level_7", "Slide"], ["Step Resolution8", "Ring"], ["UseMLVal_Level_8", "Slide"], ["Freq Rounding8", "Boolean"], ["Duration8(s)", "Numeric"], ["Tones8", "Numeric"], ["Rounding Val8", "Numeric"], ["Level1", "Boolean"], ["Step Progression1", "Boolean"], ["Frequency Range1", "Boolean"], ["Step Size1", "Boolean"], ["Level2", "Boolean"], ["Step Progression2", "Boolean"], ["Frequency Range2", "Boolean"], ["Frequency(Hz)3", "Boolean"], ["Step Progression3", "Boolean"], ["Level Range3", "Boolean"], ["WAV Info4", "Boolean"], ["Level4", "Boolean"], ["Instrument Settings5", "Boolean"], ["Sweep Settings5", "Boolean"], ["Level Range5", "Boolean"], ["Sweep Type6", "Boolean"], ["Level6", "Boolean"], ["Frequency Range6", "Boolean"], ["Step Size6", "Boolean"], ["Level6_1", "Boolean"], ["Fixed Ton (Hz)6", "Boolean"], ["Level7", "Boolean"], ["Noise7", "Boolean"], ["Frequency Range7", "Boolean"], ["Level8", "Boolean"], ["Multitone8", "Boolean"], ["Frequency Range8", "Boolean"], ["Stimulus Type", "Ring"], ["OK", "Boolean"], ["Cancel", "Boolean"], ["Wave Channel", "Ring"], ["StartFreq1_Caption", "String"], ["StopFreq1_Caption", "String"], ["StartFreq2_Caption", "String"], ["StopFreq2_Caption", "String"], ["StartFreq6_Caption", "String"], ["StopFreq6_Caption", "String"], ["StartFreq7_Caption", "String"], ["StopFreq7_Caption", "String"], ["StartFreq8_Caption", "String"], ["StopFreq8_Caption", "String"], ["Output Imp1", "Ring"], ["Nominal Imp1", "Numeric"], ["V on DUT1", "Boolean"], ["Output Imp2", "Ring"], ["Nominal Imp2", "Numeric"], ["V on DUT2", "Boolean"], ["Output Imp4", "Ring"], ["Nominal Imp4", "Numeric"], ["V on DUT4", "Boolean"], ["Output Imp7", "Ring"], ["Nominal Imp7", "Numeric"], ["V on DUT7", "Boolean"], ["Output Imp8", "Ring"], ["Nominal Imp8", "Numeric"], ["V on DUT8", "Boolean"]], "Vi Ref"="Vi Ref") -> ()  [unwired: 8 in]
